vi "MoD Main-Optimize - MS PK.vi"() -> ()   [LabVIEW 2015]
uses:
  <vilib>/silver_ctls/ArrayMatrixCluster/Real Matrix NI_Silver.ctl
  <vilib>/ni845x/ni845x.llb/ni845xControl.ctl
  <vilib>/DAQmx/read.llb/DAQmx Read (Analog 1D DBL NChan 1Samp).vi
  <vilib>/MakerHub/LINX/Public/Peripherals/Analog/Analog Read 1 Chan.vi
  <vilib>/MakerHub/LINX/Public/Peripherals/Analog/Analog Read N Chans.vi
  <vilib>/MakerHub/LINX/Private/Local IO/LinxAnalogRead.vi
  <vilib>/MakerHub/LINX/Public/Utilities/Check Channel.vi
  <vilib>/DAQmx/create/channels.llb/DAQmx Create Channel (AI-Voltage-Basic).vi
  <vilib>/addons/control/pid/pid.llb/PID Control Input Filter (DBL).vi
  <vilib>/DAQmx/miscellaneous.llb/DAQmx Fill In Error Info.vi
  <vilib>/MakerHub/LINX/Private/Utilties/Generate Error.vi
  <vilib>/addons/control/pid/autopid.llb/PID Online Autotuning (Relay Feedback).vi
  <vilib>/Analysis/Matrix/Numeric/Conversions/Array To Matrix - RA2.vi
  <vilib>/ni845x/ni845x.llb/NI-845x Close Device Reference.vi
  <vilib>/addons/control/pid/NI_PID_autopid.lvlib
  <vilib>/addons/control/pid/NI_PID_pid.lvlib
  <vilib>/Analysis/Matrix/NI_Matrix.lvlib
  <vilib>/MakerHub/LINX/LMH-LINX.lvlib
  <vilib>/MakerHub/LINX/Public/Peripherals/Digital/Digital Write 1 Chan.vi
  <instrlib>/Harvard Apparatus/Harvard Apparatus PHD 2000/Harvard Apparatus PHD 2000.lvlib
panel:
  out "MS Array":dbl[](array[numeric]) format="%0.2f"
  out "MS task":refnum<k21>
  out "running?":bool=TRUE
  out "new_reactor_volume":bool[](array[boolean])
  out "new_reactor_length":bool[](array[boolean])
  out "Phase_Sensor_voltage":dbl
  out "P_tot":dbl
  out "stop_xl_write":bool=TRUE
  out "Num_exp_till_pause":i32
  out "Syringe_pump?":bool=TRUE
  out "System Error":bool=TRUE
  out "error out":errorcluster
  out "Pump setpoint(ul/min) 6":dbl format="%#_13g"
  out "Pump setpoint(ul/min) 5":dbl format="%#_13g"
  out "Pump setpoint(ul/min) 4":dbl format="%#_13g"
  out "Pump setpoint(ul/min) 3":dbl format="%#_13g"
  out "Pump setpoint(ul/min) 2":dbl format="%#_13g"
  out "Pump setpoint(ul/min) 1":dbl format="%#_13g"
  out "Volume (ul) 5":dbl format="%#_13g"
  out "Volume (ul) 4":dbl format="%#_13g"
  out "Volume (ul) 3":dbl format="%#_13g"
  out "Volume (ul) 2":dbl format="%#_13g"
  out "Volume (ul) 1":dbl format="%#_13g"
  in  "tau 5":dbl format="%#_13g"
  out "tau 4":dbl format="%#_13g"
  out "tau 3":dbl format="%#_13g"
  out "tau 2":dbl format="%#_13g"
  out "tau 1":dbl format="%#_13g"
  out "Reactor Length":dbl format="%#_13g"
  out "Flowrate Sensor 2":dbl format="%#_13g"
  out "Flowrate Sensor 1":dbl format="%#_13g"
  out "Pressure 2":dbl format="%#_13g"
  out "Pressure 1":dbl format="%#_13g"
  out "Temperature Control 5":bool=TRUE
  out "Temperature Control 4":bool=TRUE
  out "Temperature Control 3":bool=TRUE
  out "Temperature Control 2":bool=TRUE
  out "Temperature Control 1":bool=TRUE
  out "Temperature SP 5":dbl format="%#_g'C"
  out "Temperature SP 4":dbl format="%#_g'C"
  out "Temperature SP 3":dbl format="%#_g'C"
  out "Temperature SP 2":dbl format="%#_g'C"
  out "Temperature SP 1":dbl format="%#_g'C"
  in  "Bay Temperature 5":dbl
  in  "SSR Duration 5":dbl
  in  "SSR Duration 4":dbl
  in  "SSR Duration 3":dbl
  in  "SSR Duration 2":dbl
  in  "SSR Duration 1":dbl
  in  "Total Product Amount":dbl=1.0 format="%#_gml"
  out "Setup Error":bool=TRUE
  out "Error Message":string
  out "ID CTR":i32
  in  "Tab Control":T1(tab)
  out "Reagent pic 5":picture
  in  "reagent name 5":string
  out "Reagent Pic 4":picture
  in  "reagent name 4":string
  out "Reagent Pic 3":picture
  in  "reagent  name 3":string
  in  "Product name":string
  in  "reagent name 1":string="2,5 hexanedione"
  out "Reagent Pic 1":picture
  in  "Vr5":dbl=45.6036 format="%#_guL"
  in  "Vr4":dbl format="%#_guL"
  in  "Vr3":dbl=45.6036 format="%#_guL"
  in  "Vr2":dbl format="%#_guL"
  in  "Vr1":dbl format="%#_guL"
  in  "System decide help Button":bool
  in  "Reaction Scheme Confirm":bool
  in  "Synthesis Route Array":string[][](array[string])=[["2,5 hexanedione", "1", "PhB(OH)2", "", "", ""], ["ethanolamine", "1", "-", "-", "-", "-"], ["", "", "-", "-", "-", "-"], ["", "", "-", "-", "-", "-"], ["", "", "-", "-", "-", "-"], ["", "", "-", "-", "-", "-"]]
  in  "System decide help Button 2":bool
  out "Setup Confirm":bool=TRUE
  in  "BAY 1":u16(ring)=1 items=["               Bypass", "         Heated Reactor", "    Small Heated Reator", "         Cooled Reactor", "      Packed Bed Reactor", "          Photo Reactor", "             Separator"]
  in  "BAY 5":u16(ring) items=["               Bypass", "         Heated Reactor", "    Small Heated Reactor", "         Cooled Reactor", "     Packed Bed Reactor", "         Photo Reactor", "             Separator"]
  in  "BAY 4":u16(ring) items=["                Bypass", "         Heated Reactor", "    Small Heated Reactor", "         Cooled Reactor", "     Packed Bed Reactor", "         Photo Reactor", "             Separator"]
  in  "BAY 3":u16(ring) items=["               Bypass", "         Heated Reactor", "    Small Heated Reactor", "         Cooled Reactor", "     Packed Bed Reactor", "          Photo Reactor", "             Separator"]
  in  "BAY 2":u16(ring) items=["               Bypass", "         Heated Reactor", "    Small Heated Reactor", "         Cooled Reactor", "      Packed Bed Reactor", "          Photo Reactor", "             Separator"]
  out "Reagent Pic 2":picture
  out "Product Pic":picture
  in  "reagent name 2":string="ethanolamine"
  in  "reagent name 6":string
  out "Reagent Pic 6":picture
  in  "System Parameters Help Button":bool
  out "Setup Confirm 2":bool
  in  "System Parameters Confirm Button":bool
  in  "Bay Parameters":T2={"Bay 1 "={"Pump 1 Flowrate"=0.0, "optimize_temp"=TRUE, "optimize_tau"=TRUE, "Run at set flowrate"=FALSE, "Pump 2 Flowrate"=0.0, "Temperature Params"=[40.0, 80.0, 100.0], "pump params 1"=[20.0, 190.0, 325.0], "pump params 2"=[20.0, 190.0, 325.0], "Temperature"=0.0, "Run at set temperature"=FALSE}, "Bay 2 "={"Pump 3 Flowrate"=0.0, "optimize_temp"=FALSE, "optimize_tau"=FALSE, "Run at set flowrate"=FALSE, "Temperature Params"=[40.0, 100.0, 100.0], "Resisdence time params"=[38.03, 347.0, 650.0], "pump_at_ratio"=FALSE, "pump_num_ratio"=0.0, "Temperature"=0.0, "Run at set temperature"=FALSE}, "Bay 3 "={"Pump 4 Flowrate"=100.0, "optimize_temp"=FALSE, "optimize_tau"=FALSE, "Run at set flowrate"=FALSE, "Temperature Params"=[40.0, 100.0, 100.0], "Resisdence time params"=[3.8, 34.7, 0.0], "pump_at_ratio"=FALSE, "pump_num_ratio"=0.2, "Temperature "=100.0, "Run at set temperature"=FALSE}, "Bay 4 "={"Pump 5 Flowrate"=40.0, "Run at set flowrate"=FALSE, "optimize_temp"=FALSE, "optimize_tau"=FALSE, "Resisdence time params"=[10.0, 50.0, 225.0], "Temperature Params"=[40.0, 100.0, 80.0], "pump_at_ratio"=FALSE, "pump_num_ratio"=1.0, "Temperature"=0.0, "Run at set temperature"=FALSE}, "Bay 5 "={"Pump 6 Flowrate"=0.0, "Run at set flowrate"=FALSE, "optimize_temp"=FALSE, "optimize_tau"=FALSE, "Resisdence time params"=[1.0, 5.0, 0.0], "Temperature Params"=[0.0, 0.0, 0.0], "pump_at_ratio"=FALSE, "pump_num_ratio"=0.5, "Temperature"=0.0, "Run at set temperature"=FALSE}, "Excel File Name"="C:\\Users\\Admin\\Dropbox (MIT)\\MoD Files\\Data\\PK_MS080917", "hplc File Name"="C:\\Chem32\\1\\Data\\MOD", "Matlab File"="C:\\Users\\Admin\\Dropbox (MIT)\\MoD Files\\Data\\PK_MS081017", "Syringe for Pump 2?"=TRUE, "Num_conditons_per_wait"=2.0, "Continue from previous optimization?"=FALSE, "Total Number of Experiments 2"=15.0, "Hplc Wait time(min)"=1.0, "increas_decrease_hplc_peak"=TRUE, "Internal Standard?"=TRUE, "ISTD start"=8.0, "ISTD end"=10.0, "hplc_start"=1.75, "hplc_end"=3.0, "throughput_yield"=FALSE} {"Hplc Wait time(min)" format="%#_13g"; "Bay 5"."Temperature Params" format="%#_g'C"; "Bay 4"."Temperature Params" format="%#_g'C"; "Bay 3"."Temperature Params" format="%#_g'C"; "Bay 2"."Temperature Params" format="%#_g'C"; "Bay 1"."Temperature Params" format="%#_g'C"}
  out "System Confirm Not Clicked":string
  out "pause for ms":bool=TRUE
  out "best_exp_num":dbl=1.0
  out "temperature_best":dbl[](array[numeric])
  out "Flowrates(ul/min)_best":dbl[](array[numeric])
  out "System Status":u16(ring)=2 caption="Sy" items=["System  Error", "System Running", "System Standby"]
  out "Current Experiment":dbl=1.0
  out "Total Number of Experiments":dbl=33.0
  out "Phase Sensor Chart":T3(graph)
  out "HPLC Analysis":bool
  out "Equlibrating Temperature":bool
  out "Flushing System":bool
  out "Calculate condition":bool
  out "Temperature 5":dbl format="%#_g'C"
  out "Temperature 4":dbl format="%#_g'C"
  out "Temperature 3":dbl format="%#_g'C"
  out "Temperature 2":dbl format="%#_g'C"
  out "Temperature 1":dbl format="%#_g'C"
  out "Flowrate Chart":T4(graph)
  out "Teperature Chart":T3(graph)
  out "Pump Setpoints Chart":T3(graph)
  out "Pressure Chart":T3(graph)
  out "Optimization_loop_index":i32
  out "curr_wait_time":dbl
  out "total_flush_time":dbl
  out "Temp SS? 5":bool=TRUE
  out "Temp SS? 4":bool=TRUE
  out "Temp SS? 3":bool=TRUE
  out "Temp SS? 2":bool=TRUE
  out "Temp SS? 1":bool=TRUE
  out "System Flushed?":bool
  out "stop_button clicked":bool
  out "MS Signals Chart":dbl[][](graph)
  in  "MS Analog Channel":tag="cDAQ1Mod1/ai0"
  out "experiment history":T5
  in  "Number of System Flushes per condtion":dbl=2.5
  in  "calculate volume 3":bool
  in  "calculate volume 2":bool=TRUE
  in  "calculate volume 1":bool=TRUE
  in  "calculate volume 4":bool
  in  "calculate volume 5":bool
  in  "Extra system dead volume":dbl format="%#_gul"
  in  "new reactor length? 1":bool
  in  "tube_length(in)":dbl[](array[numeric])=[188.0, 188.0, 10.0, 10.0, 10.0]
  out "Pause Before Analysis":bool
  out "Chiller COMM Port":bool
  out "Arduino COMM Port 2":bool
  out "Temperature Sensor COMM Port":bool
  out "Flow Rate":bool
  out "Pressure":bool
  out "Pump COMM Port":bool
  in  "COMM Port :: Milligat Pumps":refnum<visa-resource-name>="COM8"
  in  "Arduino COMM Port":refnum<visa-resource-name>="COM7"
  in  "Sample Valve COMM::Port":refnum<visa-resource-name>="COM10"
  in  "COMM Port:: Harvard Syringe Pump":refnum<visa-resource-name>="COM13"
  in  "tube_id(in)":enum16{".01", ".02", ".03", ".04"}[](array[ring])=[enum.".03", enum.".03", enum.".03", enum.".03", enum.".03"]
  out "Total System Resisdence Time(min)":dbl
  in  "Debug_run_button":bool
  in  "new reactor length? 2":bool
  in  "new reactor length? 3":bool
  in  "new reactor length? 4":bool
  in  "new reactor length? 5":bool
  in  "IR Sensor Device":T6="USB0::0x3923::0x7514::01B3FF21::RAW"
  out "Stop":bool=TRUE
  in  "Run_Stop_cluster":T7
  # "Molecules on Demand"
  # "Synthetic Route"
  # "5"
  # "6"
  # "4"
  # "Product"
  # "1"
  # "2"
  # "3"
  # "Reagent List"
  # "Concentration(M)"
  # "Molecule"
  # "1"
  # "1"
  # "2"
  # "2"
  # "3"
  # "3"
  # "4"
  # "4"
  # "5"
  # "6"
  # "5"
  # "6"
  # "Product"
  # "Reactor Volume:"
  # "Optimization Parameters"
  # "Pause after"
  # "Experiments"
  # "Optimize for"
  # "to"
  # "of HPLC Peak from"
  # "from"
  # "to"
  # "min"
  # "min"
  # "HPLC runtime"
  # "# Iterations"
  # "Reporting"
  # "Excel Output File Name"
  # "HPLC File Path"
  # "MATLAB File Path"
  # "Temperature"
  # "Flowrate(ul/min)"
  # "Lower Bound"
  # "Upper Bound"
  # "Optimize?"
  # "-or-"
  # "Run at"
  # "times incoming flow"
  # "Setpoint"
  # "Temperature"
  # "Flowrate(ul/min)"
  # "Lower Bound"
  # "Upper Bound"
  # "Optimize?"
  # "-or-"
  # "Run at"
  # "times incoming flow"
  # "Setpoint"
  # "Temperature"
  # "Flowrate(ul/min)"
  # "Lower Bound"
  # "Upper Bound"
  # "Optimize?"
  # "-or-"
  # "Run at"
  # "times incoming flow"
  # "Setpoint"
  # "Temperature"
  # "Flowrate 3 (ul/min)"
  # "Lower Bound"
  # "Upper Bound"
  # "Optimize?"
  # "-or-"
  # "Run at"
  # "times incoming flow"
  # "Setpoint"
  # "Temperature"
  # "Flowrate 1(ul/min)"
  # "Flowrate 2(ul/min)"
  # "Lower Bound"
  # "Upper Bound"
  # "Optimize?"
  # "Setpoint"
  # "Pressure (psi)"
  # "System Status"
  # "Temperature('C)"
  # "BAY"
  # "1"
  # "2"
  # "3"
  # "4"
  # "5"
  # "Pump Flowrate Setpoint(ul/min)"
  # "Flowrate (ul/min)"
  # "Phase Sensor"
  # "Current Experiment"
  # "MS Chart"
  # "Temperature('C)"
  # "Flowrate(ul/min)"
  # "Exp"
  # "Current Best Condition"
  # "Time to reach steady state:"
  # "Current Wait Time:"
  # "Experimental Steps"
  # "Calculated New Conditions"
  # "Steady State"
  # "Analyzed HPLC"
  # "Equilibrated Temperature"
  # "Tube Length (cm)"
  # "Bay"
  # "Tube ID (in)"
  # "Calculate Volume"
  # "Use new tube length"
  # "1."
  # "2."
  # "3."
  # "4."
  # "5."
  # "Reactor Lengths\n*Heated Reactor - 188cm * Small Reactor - 99cm * Bypass - 10cm * Separator - *"
  # "All Experimental Data"
  # "P1"
  # "P2"
  # "P3"
  # "P4"
  # "P5"
  # "P6"
  # "T1"
  # "T2"
  # "T3"
  # "T4"
  # "T5"
  # "Obj_fun"
  # "HPLC_Data"
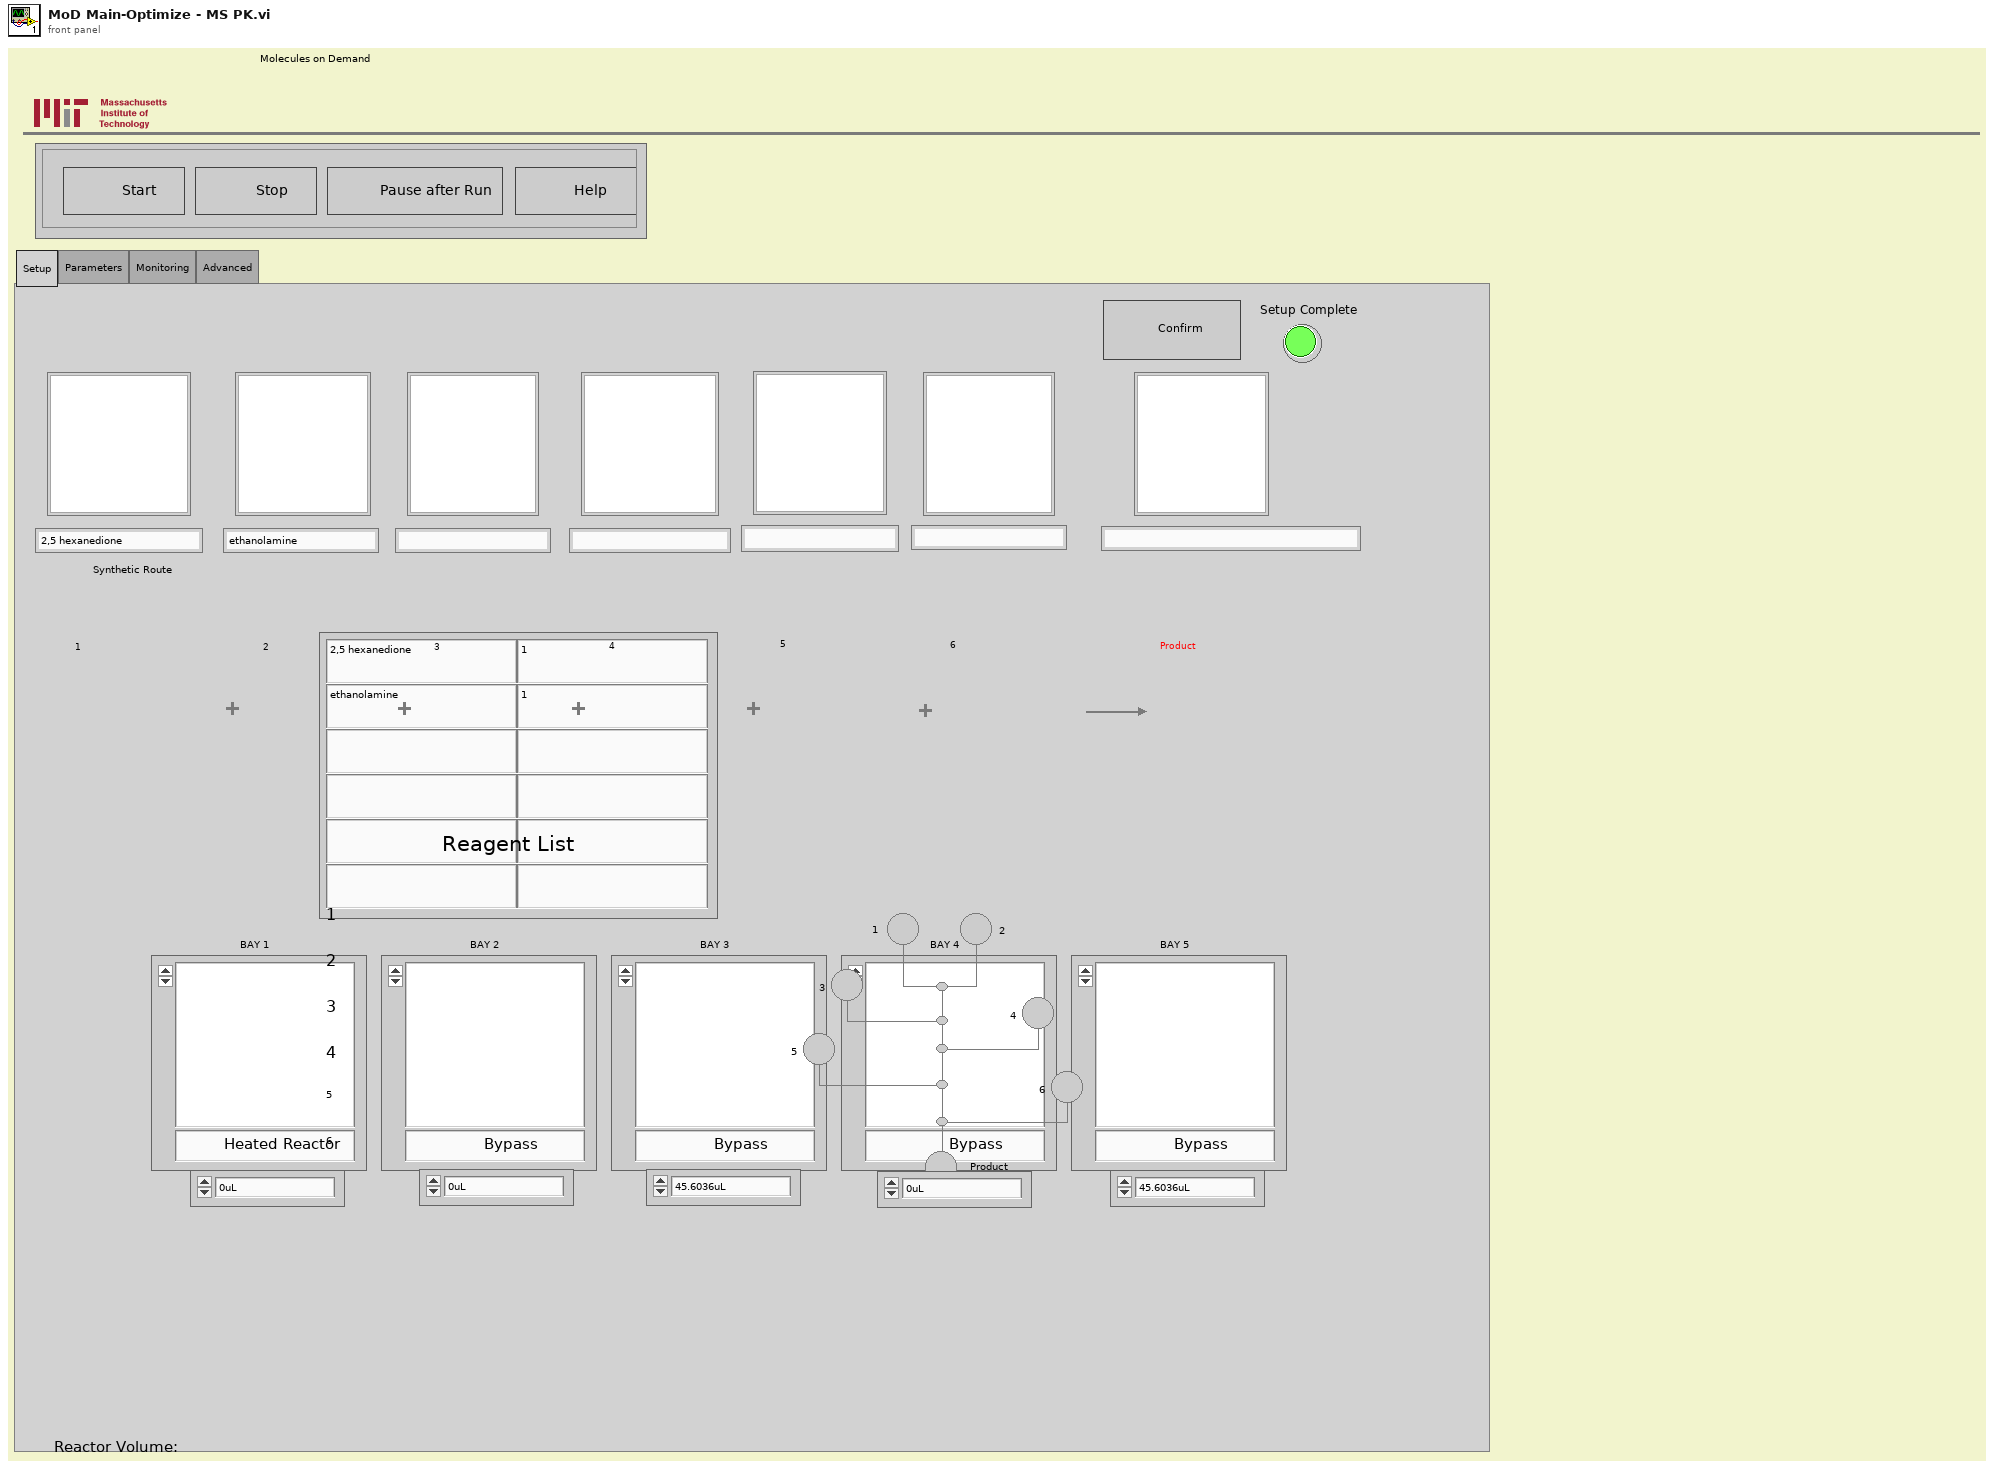
[diagram p1: front panel]
types:
  T1 = enum32{"Setup", "Parameters", "Monitoring", "Advanced"}
  T2 = cluster{"Bay 1 ":cluster{"Pump 1 Flowrate":dbl, "optimize_temp":bool, "optimize_tau":bool, "Run at set flowrate":bool, "Pump 2 Flowrate":dbl, "Temperature Params":dbl[], "pump params 1":dbl[], "pump params 2":dbl[], "Temperature":dbl, "Run at set temperature":bool}, "Bay 2 ":cluster{"Pump 3 Flowrate":dbl, "optimize_temp":bool, "optimize_tau":bool, "Run at set flowrate":bool, "Temperature Params":dbl[], "Resisdence time params":dbl[], "pump_at_ratio":bool, "pump_num_ratio":dbl, "Temperature":dbl, "Run at set temperature":bool}, "Bay 3 ":cluster{"Pump 4 Flowrate":dbl, "optimize_temp":bool, "optimize_tau":bool, "Run at set flowrate":bool, "Temperature Params":dbl[], "Resisdence time params":dbl[], "pump_at_ratio":bool, "pump_num_ratio":dbl, "Temperature ":dbl, "Run at set temperature":bool}, "Bay 4 ":cluster{"Pump 5 Flowrate":dbl, "Run at set flowrate":bool, "optimize_temp":bool, "optimize_tau":bool, "Resisdence time params":dbl[], "Temperature Params":dbl[], "pump_at_ratio":bool, "pump_num_ratio":dbl, "Temperature":dbl, "Run at set temperature":bool}, "Bay 5 ":cluster{"Pump 6 Flowrate":dbl, "Run at set flowrate":bool, "optimize_temp":bool, "optimize_tau":bool, "Resisdence time params":dbl[], "Temperature Params":dbl[], "pump_at_ratio":bool, "pump_num_ratio":dbl, "Temperature":dbl, "Run at set temperature":bool}, "Excel File Name":string, "hplc File Name":string, "Matlab File":string, "Syringe for Pump 2?":bool, "Num_conditons_per_wait":dbl, "Continue from previous optimization?":bool, "Total Number of Experiments 2":dbl, "Hplc Wait time(min)":dbl, "increas_decrease_hplc_peak":bool, "Internal Standard?":bool, "ISTD start":dbl, "ISTD end":dbl, "hplc_start":dbl, "hplc_end":dbl, "throughput_yield":bool}
  T3 = cluster{"[0]":dbl, "[1]":dbl, "[2]":dbl, "[3]":dbl, "[4]":dbl, "[5]":dbl, "[6]":dbl, "[7]":dbl, "[8]":dbl}
  T4 = cluster{"[0]":i32, "[1]":i32, "[2]":i32, "[3]":i32, "[4]":i32, "[5]":i32, "[6]":i32, "[7]":i32, "[8]":i32}
  T5 = typedef "Real Matrix NI_Silver.ctl" = dbl[][]
  T6 = typedef "ni845xControl.ctl" = refnum<k21>
  T7 = cluster{"Stop":bool, "Run":bool, "Stop Run Button":bool, "Help Button":bool}
  T8 = cluster{"Proportional gain Kc":dbl, "Integral time Ti (sec)":dbl, "Derivative time Ti (sec)":dbl}
  T9 = cluster{"type of controller":enum16{"P", "PI", "PID"}, "relay cycles":i32, "relay amplitude":dbl, "control specifications":enum16{"Fast", "Normal", "Slow"}, "PV noise level":dbl}
  T10 = typedef "LMH-LINX.lvlib/LINX Ref.ctl" = cluster{"IO":T11, "Interface":T12, "LINX Device Config":T13}
  T11 = typedef "LMH-LINX.lvlib/Platform.ctl" = enum16{"Remote", "Local"}
  T12 = typedef "LMH-LINX.lvlib/Interface.ctl" = enum16{"Serial", "TCP"}
  T13 = typedef "LMH-LINX.lvlib/Device.lvlib/LINX Device Config.ctl" = cluster{"Interface":T12, "COM Port":refnum<visa-resource-name>, "TCP Configuration":T14, "Device Family":u8, "Device ID":u8, "Device Name":string, "TCP Ref":refnum<k5>, "Channels":T15}
  T14 = typedef "LMH-LINX.lvlib/Device.lvlib/TCP Config.ctl" = cluster{"IP Address":string, "Port":u16}
  T15 = typedef "LMH-LINX.lvlib/Channels.ctl" = cluster{"DI":u8[], "DO":u8[], "AI":u8[], "AO":u8[], "PWM":u8[], "QE":u8[], "UART":u8[], "I2C 2":u8[], "SPI":u8[], "CAN":u8[], "Servo":u8[], "AI Ref (V)":dbl, "AI Resolution (Bits)":u8, "AO Ref (V)":dbl, "AO Resolution (Bits)":u8}
  T16 = typedef "imagedata.ctl" = cluster{"image type":i32, "image depth":i32, "image":u8[], "mask":u8[], "colors":u32[], "Rectangle":cluster{"left":i16, "top":i16, "right":i16, "bottom":i16}}
  T17 = cluster{"proportional gain (Kc)":dbl, "integral time (Ti, min)":dbl, "derivative time (Td, min)":dbl}
  T18 = typedef "NI_Matrix.lvlib/RealMatrix.ctl" = dbl[][]
  T19 = enum16{"Left Button", "Center Button", "Right Button", "Window Close"}
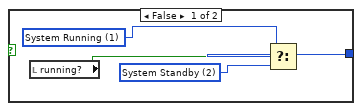
[diagram p3: hidden frame]
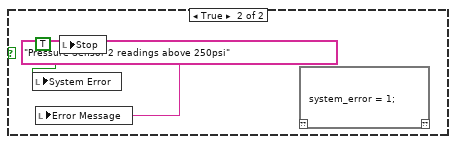
[diagram p4: hidden frame]
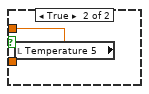
[diagram p6: hidden frame]
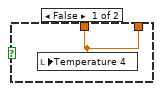
[diagram p7: hidden frame]
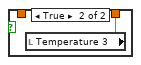
[diagram p8: hidden frame]
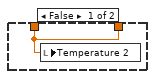
[diagram p9: hidden frame]
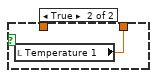
[diagram p10: hidden frame]
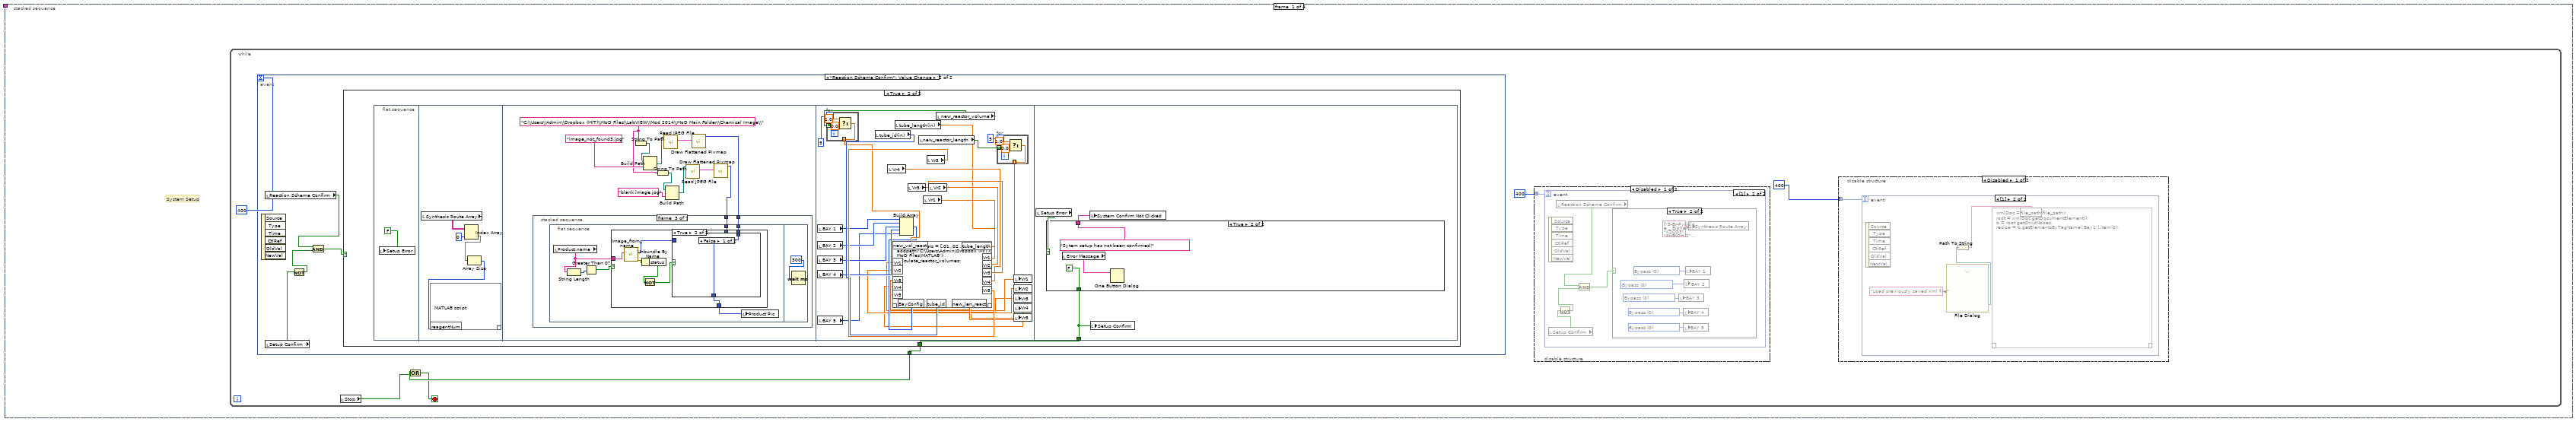
[diagram p11: hidden frame]
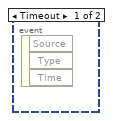
[diagram p12: hidden frame]
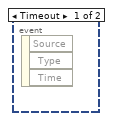
[diagram p14: hidden frame]
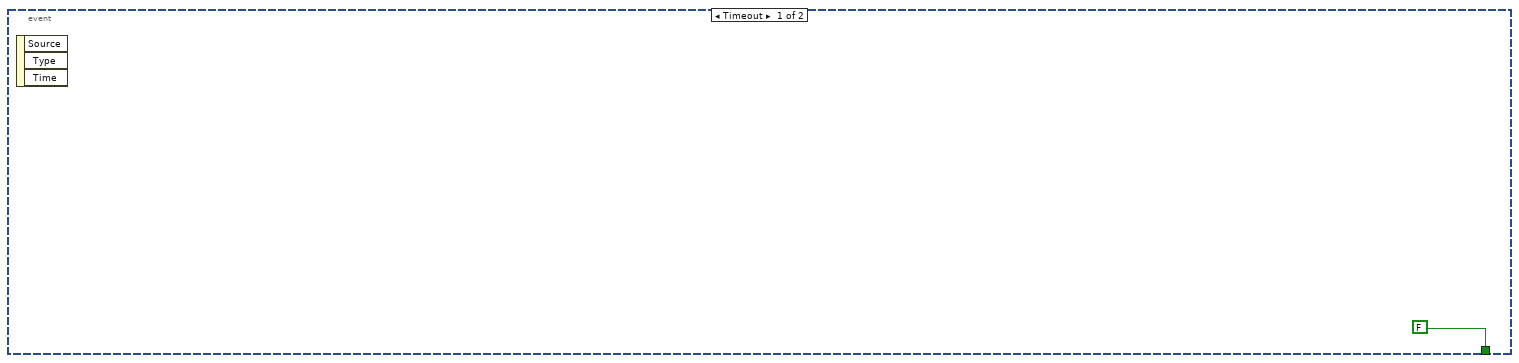
[diagram p17: hidden frame]
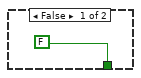
[diagram p18: hidden frame]
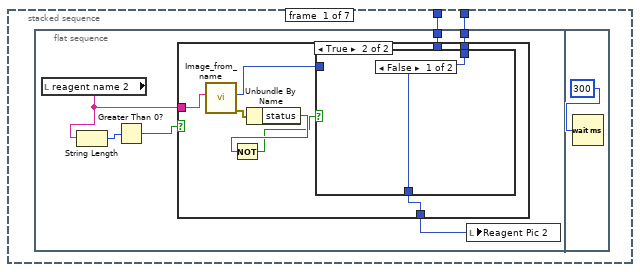
[diagram p19: hidden frame]
diagram:
  # "Assume User always uses the first bay first"
  n1 = flat-sequence {
    tunnel: ["COMM Port :: Milligat Pumps"] -> w9
    tunnel: ["Arduino COMM Port"] -> w8
    tunnel: [w13] -> w5
    tunnel: ["Bay Parameters"] -> w4
    tunnel: [w61] -> w10
    tunnel: w9 -> [w61]
    tunnel: w8 -> [w49]
    tunnel: [w55] -> w7
    tunnel: [w53] -> w6
    tunnel: w5 -> [w53]
    tunnel: w4 -> [w51]
    tunnel: [w48] -> w3
    tunnel: w10 -> [w67]
    tunnel: w7 -> [w66]
    tunnel: w6 -> [w64]
    tunnel: w3 -> [w62]
    tunnel: [w62] -> w1
    tunnel: [w1358] -> w2
    tunnel: w1 -> [w1358]
    tunnel: w2 -> [w1359]
    frame #0 {
      w37 = FALSE ("Equlibrating Temperature")
      n2 = call-poly <vilib>:"DAQmx Create Virtual Channel.vi"("physical channels"="MS Analog Channel") -> ("task out"=→"MS task":refnum<k21>)  [unwired: 13 in, 1 out]
      n3 = script code="TempArr1=[23 23 23 23 23 23 23 23 23 23]';\nTempArr2=[23 23 23 23 23 23 23 23 23 23]';\nTempArr3=[23 23 23 23 23 23 23 23 23 23]';\nTempArr4=[23 23 23 23 23 23 23 23 23 23]';\nTempArr5=[23 23 23 23 23 23 23 23 23 23]';\ntemp_error1 =0;\ntemp_error2 =0;\ntemp_error3 =0;\ntemp_error4 =0;\ntemp_error5 =0;\ntemp_check1 = 0;\ntemp_check2 = 0;\ntemp_check3 = 0;\ntemp_check4 = 0;\ntemp_check5 = 0;\nT1=23;\nT2=23;\nT3=23;\nT4=23;\nT5=23;"() -> ()  [unwired: 1 in, 1 out]
      n4 = Build Array("calculate volume 1", "calculate volume 2", "calculate volume 3", "calculate volume 4", "calculate volume 5") -> (→"new_reactor_volume":bool[])
      n5 = Build Array("new reactor length? 1", "new reactor length? 2", "new reactor length? 3", "new reactor length? 4", "new reactor length? 5") -> (→"new_reactor_length":bool[])
      n6 = call <vilib>:"Initialize.vi"("VISA IN"="COMM Port:: Harvard Syringe Pump") -> ("VISA OUT"=w13:refnum<visa-resource-name>)  [unwired: 13 in, 1 out]
      "Stop" <- FALSE ("Stop")
      "ID CTR" <- 0
      "Setup Confirm" <- FALSE ("Setup Confirm")
      "Error Message" <- "System shutdown sucessfully. No errors to report." ("Error Message")
      "Setup Error" <- FALSE ("Setup Error")
      "Reactor Length" <- 10.5
      "System Error" <- FALSE ("System Error")
      "Num_exp_till_pause" <- 0 ("Num_exp_till_pause")
      "Equlibrating Temperature" <- w37
      "Calculate condition" <- w37
      "Flushing System" <- w37
      "HPLC Analysis" <- w37
      "stop_xl_write" <- FALSE ("stop_xl_write")
      "Pump setpoint(ul/min) 1" <- 0.0 ("Pump setpoint(ul/min) 1")
      "Pump setpoint(ul/min) 2" <- 0.0 ("Pump setpoint(ul/min) 2")
      "Pump setpoint(ul/min) 4" <- 0.0 ("Pump setpoint(ul/min) 4")
      "Pump setpoint(ul/min) 6" <- 0.0 ("Pump setpoint(ul/min) 6")
      "Pump setpoint(ul/min) 3" <- 0.0 ("Pump setpoint(ul/min) 3")
      "Pump setpoint(ul/min) 5" <- 0.0 ("Pump setpoint(ul/min) 5")
      "Setup Confirm 2" <- FALSE ("Setup Confirm 2")
      "running?" <- FALSE ("running?")
    }
    frame #1 {
      w50 = FALSE
      w60 = 23
      (unwired) path "C:/Users/User1/Documents/Lab/MoD/Images"
      n7 = disable-structure shown="Disabled" {
        frame Disabled {
          n8 = local read "BAY 2"() -> ()  [unwired: 1 out]
          n9 = local read "BAY 3"() -> ()  [unwired: 1 out]
          n10 = local read "BAY 4"() -> ()  [unwired: 1 out]
          n11 = local read "BAY 5"() -> ()  [unwired: 1 out]
          n12 = local read "BAY 1"() -> ()  [unwired: 1 out]
        }
        frame Enabled {
        }
      }
      n13 = local write "Debug_run_button"(TRUE) -> ()
      n14 = call <vilib>:"Initialize.vi"("Serial Port"=w49) -> ("LINX Resource"=w48:T10)  [unwired: 8 in, 2 out]
      n15 = local write "System Parameters Confirm Button"(w50) -> ()
      n16 = local write "Setup Confirm 2"(w50) -> ()
      n17 = Unbundle By Name(w51) -> ("Syringe for Pump 2?"=→"Syringe_pump?":bool)
      n18 = local write "Temperature 1"(w60) -> ()
      n19 = local write "Temperature 2"(w60) -> ()
      n20 = local write "Temperature 3"(w60) -> ()
      n21 = local write "Temperature 4"(w60) -> ()
      n22 = local write "Temperature 5"(w60) -> ()
      n23 = local write "Temperature SP 1"(w60) -> ()
      n24 = local write "Temperature SP 2"(w60) -> ()
      n25 = local write "Temperature SP 3"(w60) -> ()
      n26 = local write "Temperature SP 4"(w60) -> ()
      n27 = local write "Temperature SP 5"(w60) -> ()
      n28 = Current VI's Path() -> (path=w59:path)
      n29 = Strip Path(path=w59) -> (stripped path=w57:path)  [unwired: 1 out]
      n30 = Strip Path(path=w57) -> (stripped path=w56:path)  [unwired: 1 out]
      n31 = Build Path(base path=w56, name or relative path="MATLAB") -> (appended path=w55:path)
    }
    frame #2 {
      # "Main Help Dialog Popup"
      n32 = while {
        stop <- w1352 stop-if-true
        n33 = event shown="[6] \"Run_Stop_cluster.Run\": Value Change" {
          selector: _ -> [_ _ _ _ _ _ _]
          dyn-events: _ -> [_ _ _ _ _ _ _]
          timeout: 100 -> [_ _ _ _ _ _ _]
          event Timeout {
            n34 = event-data() -> ()  [unwired: 1 in, 3 out]
          }
          event "Run_Stop_cluster.Help Button": Value Change {
            n35 = local read "Run_Stop_cluster"() -> (w1355:T7)
            n36 = event-data() -> ()  [unwired: 1 in, 4 out]
            n37 = Unbundle By Name(w1355) -> ("Help Button"=w1354:bool)
            n38 = case shown="True" w1354 {
              frame False {
              }
              frame True {
                n39 = call "help.vi"() -> ()  [unwired: 11 in]
              }
            }
          }
          event "System decide help Button": Value Change {
            n40 = event-data() -> ()  [unwired: 1 in, 5 out]
            n41 = call "help_synthesis_man-auto_instructions.vi"() -> ()  [unwired: 12 in]
          }
          event "System Parameters Help Button": Value Change {
            n42 = event-data() -> ()  [unwired: 1 in, 5 out]
            n43 = call "help_parameters_setup.vi"() -> ()  [unwired: 12 in]
          }
          event "System decide help Button 2": Value Change {
            n44 = event-data() -> ()  [unwired: 1 in, 5 out]
            n45 = call "help_synthesis_route_instructions.vi"() -> ()  [unwired: 12 in]
          }
          event "Run_Stop_cluster.Stop": Value Change {
            n46 = event-data() -> ()  [unwired: 1 in, 5 out]
            n47 = local write "Stop"(TRUE) -> ()
          }
          event "Run_Stop_cluster.Run": Value Change {
            n48 = event-data() -> ()  [unwired: 1 in, 5 out]
            n49 = local write "running?"(TRUE) -> ()
          }
        }
        n50 = local read "Stop"() -> (w1352:bool)
      }
      n51 = stacked-sequence {
        tunnel: w67 -> [_ _ _ _]
        tunnel: w66 -> [_ w431 _ _]
        tunnel: w64 -> [_ _ _ w598]
        tunnel: w62 -> [_ _ _ w596]
        frame #0 {
          # "System Setup"
          n52 = while {
            stop <- w206 stop-if-true
            n53 = event shown="[1] \"Reaction Scheme Confirm\": Value Change" {
              selector: _ -> [_ _]
              dyn-events: _ -> [_ _]
              timeout: 400 -> [_ _]
              tunnel: [FALSE w226] -> w208
              event Timeout {
                n54 = event-data() -> ()  [unwired: 1 in, 3 out]
              }
              event "Reaction Scheme Confirm": Value Change {
                n55 = event-data() -> ()  [unwired: 1 in, 6 out]
                n56 = local read "Reaction Scheme Confirm"() -> (w230:bool)
                n57 = local read "Setup Confirm"() -> (w228:bool)
                n58 = Not(x=w228) -> (.not. x?=w227:bool)
                n59 = And(x=w230, y=w227) -> (x .and. y?=w229:bool)
                n60 = case shown="True" w229 {
                  tunnel: [FALSE w232] -> w226
                  frame False {
                  }
                  frame True {
                    n61 = flat-sequence {
                      tunnel: [w421] -> w232
                      frame #0 {
                        n62 = local write "Setup Error"(FALSE) -> ()
                      }
                      frame #1 {
                        n63 = local read "Synthesis Route Array"() -> (w236:string[][])
                        n64 = Index Array(array=w236, index (col)=0 ("disabled index (col)")) -> (element=w234:string[])  [unwired: 1 in]
                        n65 = Array Size(array=w234) -> (size(s)=w237:i32)
                        n66 = script code="MATLAB script"("reagentNum"=w237) -> ()  [unwired: 1 in, 1 out]
                      }
                      frame #2 {
                        w240 = "C:\\Users\\Admin\\Dropbox (MIT)\\MoD Files\\LabVIEW\\Mod 2014\\MoD Main Folder\\Chemical Image\\" ("string")
                        n67 = String To Path(string=w240) -> (path=w246:path)
                        n68 = Build Path(base path=w246, name or relative path="image_not_found3.jpg") -> (appended path=w245:path)
                        n69 = String To Path(string=w240) -> (path=w243:path)
                        n70 = call <vilib>:"Read JPEG File.vi"("path to JPEG file"=w245) -> ("image data"=w248:T16)  [unwired: 1 in, 9 out]
                        n71 = Build Path(base path=w243, name or relative path="blank image.jpg") -> (appended path=w241:path)
                        n72 = call <vilib>:"Read JPEG File.vi"("path to JPEG file"=w241) -> ("image data"=w244:T16)  [unwired: 1 in, 9 out]
                        n73 = call <vilib>:"Draw Flattened Pixmap.vi"("image data"=w248) -> ("new picture"=w239:picture)  [unwired: 3 in, 5 out]
                        n74 = call <vilib>:"Draw Flattened Pixmap.vi"("image data"=w244) -> ("new picture"=w238:picture)  [unwired: 3 in, 5 out]
                        n75 = stacked-sequence {
                          tunnel: w239 -> [w250 w270 w290 w310 w330 w349 w369]
                          tunnel: w238 -> [w249 w269 w289 w309 w329 w350 w370]
                          frame #0 {
                            n76 = flat-sequence {
                              tunnel: w250 -> [w256]
                              tunnel: w249 -> [w254]
                              frame #0 {
                                n77 = local read "reagent name 2"() -> (w252:string)
                                n78 = String Length(string=w252) -> (length=w255:i32)
                                n79 = Greater Than 0?(x=w255) -> (x > 0?=w253:bool)
                                n80 = case shown="True" w253 {
                                tunnel: w256 -> [_ w262]
                                tunnel: w254 -> [w257 _]
                                tunnel: [w257 w261] -> w251
                                tunnel: w252 -> [_ w260]
                                frame False {
                                }
                                frame True {
                                n81 = call "Image_from_name.vi"("Chemical Name"=w260) -> ("error out"=w263:errorcluster, "Downloaded Picture"=w264:picture)  [unwired: 8 in, 1 out]
                                n82 = Unbundle By Name(w263) -> ("status"=w259:bool)
                                n83 = Not(x=w259) -> (.not. x?=w258:bool)
                                n84 = case shown="False" w258 {
                                tunnel: w264 -> [_ w267]
                                tunnel: [w265 w266] -> w261
                                tunnel: w262 -> [w265 _]
                                frame False {
                                }
                                frame True {
                                n85 = call <vilib>:"Draw Flattened Pixmap.vi"("picture"=w267) -> ("new picture"=w266:picture)  [unwired: 8 in]
                                }
                                }
                                }
                                }
                                n86 = local write "Reagent Pic 2"(w251) -> ()
                              }
                              frame #1 {
                                n87 = Wait (ms)(milliseconds to wait=300) -> ()  [unwired: 1 out]
                              }
                            }
                          }
                          frame #1 {
                            n88 = flat-sequence {
                              tunnel: w270 -> [w276]
                              tunnel: w269 -> [w274]
                              frame #0 {
                                n89 = local read "reagent name 1"() -> (w271:string)
                                n90 = String Length(string=w271) -> (length=w275:i32)
                                n91 = Greater Than 0?(x=w275) -> (x > 0?=w273:bool)
                                n92 = case shown="True" w273 {
                                tunnel: w276 -> [_ w282]
                                tunnel: w274 -> [w277 _]
                                tunnel: [w277 w281] -> w272
                                tunnel: w271 -> [_ w280]
                                frame False {
                                }
                                frame True {
                                n93 = call "Image_from_name.vi"("Chemical Name"=w280) -> ("error out"=w283:errorcluster, "Downloaded Picture"=w284:picture)  [unwired: 8 in, 1 out]
                                n94 = Unbundle By Name(w283) -> ("status"=w279:bool)
                                n95 = Not(x=w279) -> (.not. x?=w278:bool)
                                n96 = case shown="True" w278 {
                                tunnel: w284 -> [_ w287]
                                tunnel: [w285 w286] -> w281
                                tunnel: w282 -> [w285 _]
                                frame False {
                                }
                                frame True {
                                n97 = call <vilib>:"Draw Flattened Pixmap.vi"("picture"=w287) -> ("new picture"=w286:picture)  [unwired: 8 in]
                                }
                                }
                                }
                                }
                                n98 = local write "Reagent Pic 1"(w272) -> ()
                              }
                              frame #1 {
                                n99 = Wait (ms)(milliseconds to wait=300) -> ()  [unwired: 1 out]
                              }
                            }
                          }
                          frame #2 {
                            n100 = flat-sequence {
                              tunnel: w290 -> [w296]
                              tunnel: w289 -> [w294]
                              frame #0 {
                                n101 = local read "Product name"() -> (w291:string)
                                n102 = String Length(string=w291) -> (length=w295:i32)
                                n103 = Greater Than 0?(x=w295) -> (x > 0?=w293:bool)
                                n104 = case shown="True" w293 {
                                tunnel: w296 -> [_ w302]
                                tunnel: w294 -> [w297 _]
                                tunnel: [w297 w301] -> w292
                                tunnel: w291 -> [_ w300]
                                frame False {
                                }
                                frame True {
                                n105 = call "Image_from_name.vi"("Chemical Name"=w300) -> ("error out"=w303:errorcluster, "Downloaded Picture"=w304:picture)  [unwired: 8 in, 1 out]
                                n106 = Unbundle By Name(w303) -> ("status"=w298:bool)
                                n107 = Not(x=w298) -> (.not. x?=w299:bool)
                                n108 = case shown="False" w299 {
                                tunnel: w304 -> [_ w307]
                                tunnel: [w305 w306] -> w301
                                tunnel: w302 -> [w305 _]
                                frame False {
                                }
                                frame True {
                                n109 = call <vilib>:"Draw Flattened Pixmap.vi"("picture"=w307) -> ("new picture"=w306:picture)  [unwired: 8 in]
                                }
                                }
                                }
                                }
                                n110 = local write "Product Pic"(w292) -> ()
                              }
                              frame #1 {
                                n111 = Wait (ms)(milliseconds to wait=300) -> ()  [unwired: 1 out]
                              }
                            }
                          }
                          frame #3 {
                            n112 = flat-sequence {
                              tunnel: w310 -> [w316]
                              tunnel: w309 -> [w314]
                              frame #0 {
                                n113 = local read "reagent name 6"() -> (w311:string)
                                n114 = String Length(string=w311) -> (length=w315:i32)
                                n115 = Greater Than 0?(x=w315) -> (x > 0?=w313:bool)
                                n116 = case shown="True" w313 {
                                tunnel: w316 -> [_ w322]
                                tunnel: w314 -> [w317 _]
                                tunnel: [w317 w321] -> w312
                                tunnel: w311 -> [_ w320]
                                frame False {
                                }
                                frame True {
                                n117 = call "Image_from_name.vi"("Chemical Name"=w320) -> ("error out"=w323:errorcluster, "Downloaded Picture"=w324:picture)  [unwired: 8 in, 1 out]
                                n118 = Unbundle By Name(w323) -> ("status"=w318:bool)
                                n119 = Not(x=w318) -> (.not. x?=w319:bool)
                                n120 = case shown="False" w319 {
                                tunnel: w324 -> [_ w327]
                                tunnel: [w325 w326] -> w321
                                tunnel: w322 -> [w325 _]
                                frame False {
                                }
                                frame True {
                                n121 = call <vilib>:"Draw Flattened Pixmap.vi"("picture"=w327) -> ("new picture"=w326:picture)  [unwired: 8 in]
                                }
                                }
                                }
                                }
                                n122 = local write "Reagent Pic 6"(w312) -> ()
                              }
                              frame #1 {
                                n123 = Wait (ms)(milliseconds to wait=300) -> ()  [unwired: 1 out]
                              }
                            }
                          }
                          frame #4 {
                            n124 = flat-sequence {
                              tunnel: w330 -> [w336]
                              tunnel: w329 -> [w334]
                              frame #0 {
                                n125 = local read "reagent name 5"() -> (w331:string)
                                n126 = String Length(string=w331) -> (length=w335:i32)
                                n127 = Greater Than 0?(x=w335) -> (x > 0?=w333:bool)
                                n128 = case shown="True" w333 {
                                tunnel: w336 -> [_ w342]
                                tunnel: w334 -> [w337 _]
                                tunnel: [w337 w341] -> w332
                                tunnel: w331 -> [_ w340]
                                frame False {
                                }
                                frame True {
                                n129 = call "Image_from_name.vi"("Chemical Name"=w340) -> ("error out"=w343:errorcluster, "Downloaded Picture"=w344:picture)  [unwired: 8 in, 1 out]
                                n130 = Unbundle By Name(w343) -> ("status"=w338:bool)
                                n131 = Not(x=w338) -> (.not. x?=w339:bool)
                                n132 = case shown="False" w339 {
                                tunnel: w344 -> [_ w347]
                                tunnel: [w345 w346] -> w341
                                tunnel: w342 -> [w345 _]
                                frame False {
                                }
                                frame True {
                                n133 = call <vilib>:"Draw Flattened Pixmap.vi"("picture"=w347) -> ("new picture"=w346:picture)  [unwired: 8 in]
                                }
                                }
                                }
                                }
                                n134 = local write "Reagent pic 5"(w332) -> ()
                              }
                              frame #1 {
                                n135 = Wait (ms)(milliseconds to wait=300) -> ()  [unwired: 1 out]
                              }
                            }
                          }
                          frame #5 {
                            n136 = flat-sequence {
                              tunnel: w350 -> [w354]
                              tunnel: w349 -> [w353]
                              frame #0 {
                                n137 = local read "reagent name 4"() -> (w351:string)
                                n138 = String Length(string=w351) -> (length=w356:i32)
                                n139 = Greater Than 0?(x=w356) -> (x > 0?=w355:bool)
                                n140 = case shown="True" w355 {
                                tunnel: w353 -> [_ w362]
                                tunnel: w354 -> [w357 _]
                                tunnel: [w357 w361] -> w352
                                tunnel: w351 -> [_ w360]
                                frame False {
                                }
                                frame True {
                                n141 = call "Image_from_name.vi"("Chemical Name"=w360) -> ("error out"=w363:errorcluster, "Downloaded Picture"=w364:picture)  [unwired: 8 in, 1 out]
                                n142 = Unbundle By Name(w363) -> ("status"=w358:bool)
                                n143 = Not(x=w358) -> (.not. x?=w359:bool)
                                n144 = case shown="False" w359 {
                                tunnel: w364 -> [_ w367]
                                tunnel: [w365 w366] -> w361
                                tunnel: w362 -> [w365 _]
                                frame False {
                                }
                                frame True {
                                n145 = call <vilib>:"Draw Flattened Pixmap.vi"("picture"=w367) -> ("new picture"=w366:picture)  [unwired: 8 in]
                                }
                                }
                                }
                                }
                                n146 = local write "Reagent Pic 4"(w352) -> ()
                              }
                              frame #1 {
                                n147 = Wait (ms)(milliseconds to wait=300) -> ()  [unwired: 1 out]
                              }
                            }
                          }
                          frame #6 {
                            n148 = flat-sequence {
                              tunnel: w370 -> [w374]
                              tunnel: w369 -> [w373]
                              frame #0 {
                                n149 = local read "reagent  name 3"() -> (w371:string)
                                n150 = String Length(string=w371) -> (length=w376:i32)
                                n151 = Greater Than 0?(x=w376) -> (x > 0?=w375:bool)
                                n152 = case shown="True" w375 {
                                tunnel: w373 -> [_ w382]
                                tunnel: w374 -> [w377 _]
                                tunnel: [w377 w381] -> w372
                                tunnel: w371 -> [_ w380]
                                frame False {
                                }
                                frame True {
                                n153 = call "Image_from_name.vi"("Chemical Name"=w380) -> ("error out"=w383:errorcluster, "Downloaded Picture"=w384:picture)  [unwired: 8 in, 1 out]
                                n154 = Unbundle By Name(w383) -> ("status"=w378:bool)
                                n155 = Not(x=w378) -> (.not. x?=w379:bool)
                                n156 = case shown="False" w379 {
                                tunnel: w384 -> [_ w387]
                                tunnel: [w385 w386] -> w381
                                tunnel: w382 -> [w385 _]
                                frame False {
                                }
                                frame True {
                                n157 = call <vilib>:"Draw Flattened Pixmap.vi"("picture"=w387) -> ("new picture"=w386:picture)  [unwired: 8 in]
                                }
                                }
                                }
                                }
                                n158 = local write "Reagent Pic 3"(w372) -> ()
                              }
                              frame #1 {
                                n159 = Wait (ms)(milliseconds to wait=300) -> ()  [unwired: 1 out]
                              }
                            }
                          }
                        }
                      }
                      frame #3 {
                        n160 = local read "BAY 1"() -> (w399:u16)
                        n161 = local read "BAY 2"() -> (w398:u16)
                        n162 = local read "BAY 3"() -> (w397:u16)
                        n163 = local read "BAY 4"() -> (w396:u16)
                        n164 = local read "BAY 5"() -> (w395:u16)
                        n165 = local read "tube_id(in)"() -> (w406:enum16{".01", ".02", ".03", ".04"}[])
                        n166 = local read "Vr4"() -> (w409:dbl)
                        n167 = local read "tube_length(in)"() -> (w407:dbl[])
                        n168 = Build Array(w399, w398, w397, w396, w395) -> (w394:u16[])
                        n169 = local read "Vr3"() -> (w410:dbl)
                        n170 = local read "new_reactor_length"() -> (w404:bool[])
                        n171 = local read "Vr1"() -> (w412:dbl)
                        n172 = local read "Vr5"() -> (w408:dbl)
                        n173 = local read "Vr2"() -> (w411:dbl)
                        n174 = local read "new_reactor_volume"() -> (w402:bool[])
                        n175 = for {
                          N: 5 -> [_]
                          tunnel: w402 -> [w416] mode=indexing
                          tunnel: [w413] -> w400 mode=indexing
                          n176 = Select(t=1.0, s=w416, f=0.0) -> (s? t:f=w413:dbl)
                        }
                        n177 = for {
                          N: 5 -> [_]
                          tunnel: w404 -> [w420] mode=indexing
                          tunnel: [w417] -> w403 mode=indexing
                          n178 = Select(t=1.0, s=w420, f=0.0) -> (s? t:f=w417:dbl)
                        }
                        n179 = script code="tube_diameters = [.01,.02,.03,.04];\naddpath('C:\\Users\\Admin\\Dropbox (MIT)\\MoD Files\\MATLAB');\ncalculate_reactor_volumes;"("BayConfig"=w394, "Vr1"=w412, "Vr2"=w411, "Vr3"=w410, "Vr4"=w409, "Vr5"=w408, "tube_length"=w407, "tube_id"=w406, "new_len_react"=w403, "new_vol_react"=w400) -> ("Vr1"=w393:dbl, "Vr2"=w392:dbl, "Vr3"=w391:dbl, "Vr4"=w390:dbl, "Vr5"=w389:dbl)  [unwired: 1 in, 1 out]
                        n180 = local write "Vr1"(w393) -> ()
                        n181 = local write "Vr2"(w392) -> ()
                        n182 = local write "Vr3"(w391) -> ()
                        n183 = local write "Vr4"(w390) -> ()
                        n184 = local write "Vr5"(w389) -> ()
                      }
                      frame #4 {
                        n185 = local read "Setup Error"() -> (w423:bool)
                        n186 = case shown="True" w423 {
                          tunnel: [TRUE FALSE] -> w421
                          tunnel: ["" "Sytem setup has not been confirmed!"] -> w422
                          frame False {
                          }
                          frame True {
                            n187 = local read "Error Message"() -> (w428:string)
                            n188 = One Button Dialog(message=w428) -> ()  [unwired: 1 in, 1 out]
                          }
                        }
                        n189 = local write "System Confirm Not Clicked"(w422) -> ()
                        n190 = local write "Setup Confirm"(w421) -> ()
                      }
                    }
                  }
                }
              }
            }
            n191 = local read "Stop"() -> (w207:bool)
            n192 = Or(x=w208, y=w207) -> (x .or. y?=w206:bool)
            n193 = disable-structure shown="Disabled" {
              disable-tunnel: 400 -> [w214 _]
              frame Disabled {
                n194 = event shown="[1]" {
                  selector: _ -> [_ _]
                  dyn-events: _ -> [_ _]
                  timeout: w214 -> [_ _]
                  event Timeout {
                    n195 = event-data() -> ()  [unwired: 1 in, 3 out]
                  }
                  event #1 (no event record) {
                    n196 = event-data() -> ()  [unwired: 1 in, 6 out]
                    n197 = local read "Setup Confirm"() -> (w215:bool)
                    n198 = local read "Reaction Scheme Confirm"() -> (w216:bool)
                    n199 = Not(x=w215) -> (.not. x?=w218:bool)
                    n200 = And(x=w216, y=w218) -> (x .and. y?=w217:bool)
                    n201 = case shown="True" w217 {
                      frame False {
                      }
                      frame True {
                        w220 = u16 0 items=["                     Bypass", "                Hot Reactor", "                 Separator"] ("BAY 5")
                        w221 = u16 0 items=["                     Bypass", "                Hot Reactor", "                  Separator"] ("BAY 4")
                        w222 = u16 0 items=["                     Bypass", "                 Hot Reactor", "                  Separator"] ("BAY 3")
                        w223 = u16 0 items=["                     Bypass", "                Hot Reactor", "                  Separator"] ("BAY 2")
                        w224 = u16 0 items=["                 Bypass", "             Hot Reactor", "               Separator"] ("BAY 1")
                        n202 = local write "BAY 3"(w222) -> ()
                        n203 = local write "BAY 4"(w221) -> ()
                        n204 = local write "BAY 5"(w220) -> ()
                        n205 = local write "BAY 2"(w223) -> ()
                        n206 = local write "BAY 1"(w224) -> ()
                        n207 = local write "Synthesis Route Array"(string[][] [["3-Br-Pyridine _ Biphenyl", "K2CO3", "PhB(OH)2", "", "", ""]] ("Synthesis Route Array")) -> ()
                      }
                    }
                  }
                }
              }
              frame Enabled {
              }
            }
            n208 = disable-structure shown="Disabled" {
              disable-tunnel: 400 -> [w210 _]
              frame Disabled {
                n209 = event shown="[1]" {
                  selector: _ -> [_ _]
                  dyn-events: _ -> [_ _]
                  timeout: w210 -> [_ _]
                  event Timeout {
                    n210 = event-data() -> ()  [unwired: 1 in, 3 out]
                  }
                  event #1 (no event record) {
                    n211 = event-data() -> ()  [unwired: 1 in, 6 out]
                    n212 = call "File Dialog"("prompt"="Load previously saved xml file") -> ("selected path"=w212:path)  [unwired: 11 in, 3 out]
                    n213 = Path To String(path=w212) -> (string=w211:string)
                    n214 = script code="xmlDoc = xmlread(file_path);\nroot = xmlDoc.getDocumentElement();\nb = root.getChildNodes;\nrecipe = b.getElementsByTagName('Bay1').item(0);"("file_path"=w211) -> ()  [unwired: 1 in, 1 out]
                  }
                }
              }
              frame Enabled {
              }
            }
          }
        }
        frame #1 {
          n215 = local read "Stop"() -> (w430:bool)
          n216 = Not(x=w430) -> (.not. x?=w429:bool)
          n217 = case shown="True" w429 {
            tunnel: w431 -> [_ w434]
            frame False {
              "stop_button clicked" <- TRUE ("stop_button clicked")
            }
            frame True {
              # "Parameters Initilization"
              n218 = flat-sequence {
                tunnel: w434 -> [w436]
                tunnel: [w435] -> w433
                tunnel: w433 -> [w595]
                frame #0 {
                  # "Setup bays(RFID - verify)"
                  n219 = disable-structure shown="Disabled" {
                    frame Disabled {
                      n220 = local read "BAY 1"() -> ()  [unwired: 1 out]
                      n221 = local read "BAY 2"() -> ()  [unwired: 1 out]
                      n222 = local read "BAY 3"() -> ()  [unwired: 1 out]
                      n223 = local read "BAY 4"() -> ()  [unwired: 1 out]
                      n224 = local read "BAY 5"() -> ()  [unwired: 1 out]
                    }
                    frame Enabled {
                    }
                  }
                }
                frame #1 {
                  n225 = while {
                    tunnel: w436 -> [w439]
                    tunnel: [w438] -> w435
                    stop <- w442 stop-if-true
                    n226 = flat-sequence {
                      tunnel: [w456] -> w438
                      tunnel: w439 -> [w537]
                      tunnel: [w455] -> w437
                      frame #0 {
                        n227 = while {
                          stop <- w446 stop-if-true
                          n228 = event shown="[1] \"System Parameters Confirm Button\": Value Change" {
                            selector: _ -> [_ _]
                            dyn-events: _ -> [_ _]
                            timeout: u32 200 ("milliseconds to wait") -> [_ _]
                            tunnel: [FALSE TRUE] -> w444
                            event Timeout {
                              n229 = event-data() -> ()  [unwired: 1 in, 3 out]
                            }
                            event "System Parameters Confirm Button": Value Change {
                              n230 = event-data() -> ()  [unwired: 1 in, 5 out]
                              n231 = local write "System Parameters Confirm Button"(FALSE) -> ()
                            }
                          }
                          n232 = Wait (ms)(milliseconds to wait=u32 500) -> ()  [unwired: 1 out]
                          n233 = local read "Stop"() -> (w447:bool)
                          n234 = Or(x=w447, y=w444) -> (x .or. y?=w446:bool)
                        }
                      }
                      frame #1 {
                        w476 = 0 ("disabled index (col)")
                        w488 = 1 ("disabled index (col)")
                        # "Do while parameters have not been correctly entered"
                        n235 = local read "Bay Parameters"() -> (w475:T2)
                        n236 = local read "Synthesis Route Array"() -> (w489:string[][])
                        n237 = local read "Total Number of Experiments"() -> (w508:dbl)
                        n238 = Unbundle By Name(w475) -> ("Continue from previous optimization?"=w536:bool)
                        n239 = Unbundle By Name(w475) -> ("Excel File Name"=w538:string)
                        n240 = Unbundle By Name(w475) -> ("Matlab File"=w534:string)
                        n241 = Unbundle By Name(w475) -> ("Bay 1.Run at set flowrate"=w580:bool)
                        n242 = Unbundle By Name(w475) -> ("Bay 1.Pump 1 Flowrate"=w586:dbl)
                        n243 = Unbundle By Name(w475) -> ("Bay 1.Pump 2 Flowrate"=w585:dbl)
                        n244 = Unbundle By Name(w475) -> ("Bay 2.Run at set flowrate"=w578:bool)
                        n245 = Unbundle By Name(w475) -> ("Bay 2.Pump 3 Flowrate"=w584:dbl)
                        n246 = Unbundle By Name(w475) -> ("Bay 3.Pump 4 Flowrate"=w583:dbl)
                        n247 = Unbundle By Name(w475) -> ("Bay 3.Run at set flowrate"=w577:bool)
                        n248 = Unbundle By Name(w475) -> ("Bay 4.Run at set flowrate"=w574:bool)
                        n249 = Unbundle By Name(w475) -> ("Bay 4.Pump 5 Flowrate"=w582:dbl)
                        n250 = Unbundle By Name(w475) -> ("Bay 5.Pump 6 Flowrate"=w581:dbl)
                        n251 = Unbundle By Name(w475) -> ("Bay 5.Run at set flowrate"=w573:bool)
                        n252 = Index Array(array=w489, index (row)=3, index (col)=w488) -> (element=w482:string)
                        n253 = Index Array(array=w489, index (row)=2, index (col)=w488) -> (element=w480:string)
                        n254 = Index Array(array=w489, index (row)=1, index (col)=w488) -> (element=w478:string)
                        n255 = Index Array(array=w489, index (row)=0, index (col)=w488) -> (element=w491:string)
                        n256 = Index Array(array=w489, index (row)=4, index (col)=w488) -> (element=w484:string)
                        n257 = Index Array(array=w489, index (row)=5, index (col)=w488) -> (element=w486:string)
                        n258 = Build Array(w491, w478, w480, w482, w484, w486) -> (w492:string[])
                        n259 = Index Array(array=w489, index (row)=0 ("index"), index (col)=w476) -> (element=w514:string)
                        n260 = for {
                          tunnel: w492 -> [w588] mode=indexing
                          tunnel: [w587] -> w477 mode=indexing
                          n261 = script code="ctemp1 = str2num(c_temp);"("c_temp"=w588) -> ("ctemp1"=w587:dbl)  [unwired: 1 in, 1 out]
                        }
                        n262 = Boolean To (0,1)(Boolean=w578) -> (0, 1=w533:i16)
                        n263 = Boolean To (0,1)(Boolean=w574) -> (0, 1=w575:i16)
                        n264 = Boolean To (0,1)(Boolean=w577) -> (0, 1=w576:i16)
                        n265 = Boolean To (0,1)(Boolean=w536) -> (0, 1=w535:i16)
                        n266 = Boolean To (0,1)(Boolean=w580) -> (0, 1=w579:i16)
                        n267 = Boolean To (0,1)(Boolean=w573) -> (0, 1=w572:i16)
                        n268 = Index Array(array=w489, index (row)=1 ("index"), index (col)=w476) -> (element=w509:string)
                        n269 = Index Array(array=w489, index (row)=2 ("index"), index (col)=w476) -> (element=w510:string)
                        n270 = Unbundle By Name(w475) -> ("Bay 1.optimize_temp"=w571:bool)
                        n271 = Unbundle By Name(w475) -> ("Bay 1.optimize_tau"=w569:bool)
                        n272 = Unbundle By Name(w475) -> ("Bay 2.optimize_temp"=w567:bool)
                        n273 = Unbundle By Name(w475) -> ("Bay 2.optimize_tau"=w565:bool)
                        n274 = Unbundle By Name(w475) -> ("Bay 3.optimize_temp"=w563:bool)
                        n275 = Unbundle By Name(w475) -> ("Bay 3.optimize_tau"=w561:bool)
                        n276 = Unbundle By Name(w475) -> ("Bay 4.optimize_temp"=w559:bool)
                        n277 = Unbundle By Name(w475) -> ("Bay 4.optimize_tau"=w557:bool)
                        n278 = Index Array(array=w489, index (row)=3 ("index"), index (col)=w476) -> (element=w511:string)
                        n279 = Boolean To (0,1)(Boolean=w559) -> (0, 1=w558:i16)
                        n280 = Boolean To (0,1)(Boolean=w557) -> (0, 1=w556:i16)
                        n281 = Index Array(array=w489, index (row)=4 ("index"), index (col)=w476) -> (element=w512:string)
                        n282 = Boolean To (0,1)(Boolean=w561) -> (0, 1=w560:i16)
                        n283 = Boolean To (0,1)(Boolean=w567) -> (0, 1=w566:i16)
                        n284 = Boolean To (0,1)(Boolean=w571) -> (0, 1=w570:i16)
                        n285 = Boolean To (0,1)(Boolean=w565) -> (0, 1=w564:i16)
                        n286 = Boolean To (0,1)(Boolean=w569) -> (0, 1=w568:i16)
                        n287 = Boolean To (0,1)(Boolean=w563) -> (0, 1=w562:i16)
                        n288 = Unbundle By Name(w475) -> ("Bay 5.optimize_temp"=w555:bool)
                        n289 = Unbundle By Name(w475) -> ("Bay 5.optimize_tau"=w553:bool)
                        n290 = Index Array(array=w489, index (row)=5 ("index"), index (col)=w476) -> (element=w513:string)
                        n291 = Boolean To (0,1)(Boolean=w555) -> (0, 1=w554:i16)
                        n292 = Boolean To (0,1)(Boolean=w553) -> (0, 1=w552:i16)
                        n293 = Build Array(w570, w568, w566, w564, w562, w560, w558, w556, w554, w552) -> (w551:i16[])
                        n294 = Unbundle By Name(w475) -> ("Bay 1.Temperature Params"=w548:dbl[])
                        n295 = Unbundle By Name(w475) -> ("Bay 2.Temperature Params"=w547:dbl[])
                        n296 = Unbundle By Name(w475) -> ("Bay 2.Resisdence time params"=w542:dbl[])
                        n297 = Unbundle By Name(w475) -> ("Bay 3.Temperature Params"=w546:dbl[])
                        n298 = Unbundle By Name(w475) -> ("Bay 3.Resisdence time params"=w541:dbl[])
                        n299 = Unbundle By Name(w475) -> ("Bay 4.Temperature Params"=w545:dbl[])
                        n300 = Unbundle By Name(w475) -> ("Bay 4.Resisdence time params"=w540:dbl[])
                        n301 = Unbundle By Name(w475) -> ("Bay 5.Temperature Params"=w544:dbl[])
                        n302 = Unbundle By Name(w475) -> ("Bay 5.Resisdence time params"=w539:dbl[])
                        n303 = Unbundle By Name(w475) -> ("Bay 1.pump params 2"=w507:dbl[])
                        n304 = Unbundle By Name(w475) -> ("Bay 1.pump params 1"=w543:dbl[])
                        n305 = Unbundle By Name(w475) -> ("Bay 1.Run at set temperature"=w498:bool)
                        n306 = Unbundle By Name(w475) -> ("Bay 2.Run at set temperature"=w496:bool)
                        n307 = Unbundle By Name(w475) -> ("Bay 3.Run at set temperature"=w495:bool)
                        n308 = Unbundle By Name(w475) -> ("Bay 4.Run at set temperature"=w494:bool)
                        n309 = Unbundle By Name(w475) -> ("Bay 5.Run at set temperature"=w493:bool)
                        n310 = Unbundle By Name(w475) -> ("Bay 3.Temperature"=w504:dbl)
                        n311 = Unbundle By Name(w475) -> ("Bay 1.Temperature"=w506:dbl)
                        n312 = Unbundle By Name(w475) -> ("Bay 2.Temperature"=w505:dbl)
                        n313 = Unbundle By Name(w475) -> ("Bay 4.Temperature"=w503:dbl)
                        n314 = Unbundle By Name(w475) -> ("Bay 5.Temperature"=w502:dbl)
                        n315 = Unbundle By Name(w475) -> ("Bay 3.pump_num_ratio"=w527:dbl)
                        n316 = Unbundle By Name(w475) -> ("Bay 4.pump_num_ratio"=w524:dbl)
                        n317 = Unbundle By Name(w475) -> ("Bay 5.pump_num_ratio"=w521:dbl)
                        n318 = Unbundle By Name(w475) -> ("Bay 2.pump_num_ratio"=w530:dbl)
                        n319 = Unbundle By Name(w475) -> ("Bay 4.pump_at_ratio"=w526:bool)
                        n320 = Boolean To (0,1)(Boolean=w526) -> (0, 1=w525:i16)
                        n321 = Unbundle By Name(w475) -> ("Bay 3.pump_at_ratio"=w529:bool)
                        n322 = Boolean To (0,1)(Boolean=w529) -> (0, 1=w528:i16)
                        n323 = Unbundle By Name(w475) -> ("Bay 5.pump_at_ratio"=w523:bool)
                        n324 = Boolean To (0,1)(Boolean=w523) -> (0, 1=w522:i16)
                        n325 = Unbundle By Name(w475) -> ("Bay 2.pump_at_ratio"=w532:bool)
                        n326 = Boolean To (0,1)(Boolean=w532) -> (0, 1=w531:i16)
                        n327 = Build Array(w506, w505, w504, w503, w502) -> (w501:dbl[])
                        n328 = Build Array(w498, w496, w495, w494, w493) -> (w497:bool[])
                        n329 = local read "Syringe_pump?"() -> (w454:bool)
                        n330 = for {
                          N: 5 -> [_]
                          tunnel: w497 -> [w592] mode=indexing
                          tunnel: [w591] -> w499 mode=indexing
                          n331 = Select(t=1.0, s=w592, f=0.0) -> (s? t:f=w591:dbl)
                        }
                        n332 = Unbundle By Name(w475) -> ("Internal Standard?"=w466:bool)
                        n333 = Unbundle By Name(w475) -> ("increas_decrease_hplc_peak"=w467:bool)
                        n334 = Unbundle By Name(w475) -> ("Hplc Wait time(min)"=w459:dbl)
                        n335 = Unbundle By Name(w475) -> ("Total Number of Experiments 2"=w458:dbl)
                        n336 = Unbundle By Name(w475) -> ("hplc_start"=w463:dbl)
                        n337 = Unbundle By Name(w475) -> ("ISTD start"=w461:dbl)
                        n338 = Unbundle By Name(w475) -> ("hplc_end"=w462:dbl)
                        n339 = Unbundle By Name(w475) -> ("throughput_yield"=w468:bool)
                        n340 = Unbundle By Name(w475) -> ("ISTD end"=w460:dbl)
                        n341 = Select(t=1.0, s=w454, f=0.0) -> (s? t:f=w453:dbl)
                        n342 = Select(t=1.0, s=w467, f=0.0) -> (s? t:f=w465:dbl)
                        n343 = Select(t=1.0, s=w466, f=0.0) -> (s? t:f=w464:dbl)
                        n344 = Select(t=0.0, s=w468, f=1.0) -> (s? t:f=w457:dbl)
                        n345 = script code="system_error = 0;\nnumPeaks = 1;\nstart_phase_time = 1;\nis_redo_exp = 0;\nFvalues = [];\nHPLC_Area = [];\n\nT1_span = [1 1]; T2_span = [1 1]; T3_span = [1 1]; T4_span = [1 1]; T5_span = [1 1];\nT_span = [T1_span;T2_span;T3_span;T4_span;T5_span];\n p1_span =  [1 1]; p2_span =  [1 1]; p3_span =  [1 1]; p4_span =  [1 1]; p5_span =  [1 1];  p6_span =  [1 1];\nOpt_params = [0 0 0 0 0 0 0 0 0 0 0];\nT_params = [T1_params;T2_params;T3_params;T4_params;T5_params];\npump_params = [pump1_params;pump2_params;pump3_params;pump4_params;pump5_params;pump6_params];\nopt_ctr = 0;ncall = 100;record_data = true;\nT1_SP = 23; T2_SP = 23; T3_SP = 23; T4_SP = 23; T5_SP = 23;\nT_span = [T1_span;T2_span;T3_span;T4_span;T5_span];\np_span = [p1_span;p2_span;p3_span;p4_span;p5_span;p6_span];\nno_errors = 1;\nP1 = 0; P2 =0; P3 = 0; P4 = 0; P5 = 0; P6 = 0;\nP = [P1, P2, P3,P4, P5, P6];\nis_first_set_of_exp = true;\nerror_message = 'System has no errors to report';\n%addpath(genpath('C:\\Users\\HPLC\\Dropbox (MIT)\\MoD Files\\MATLAB'))\naddpath(genpath('C:\\Users\\Admin\\Dropbox (MIT)\\MoD Files\\MATLAB'))\nallMSData = [];allHPLCData = [];allHPLCFile = [];\nBay_ratio = [0,Bay2_ratio,Bay3_ratio,Bay4_ratio,Bay5_ratio];\nBay_pump_ratio = [1, Bay2_pump_ratio, Bay3_pump_ratio, Bay4_pump_ratio, Bay5_pump_ratio];\nP_setrate = [P1_setrate, P2_setrate, P3_setrate, P4_setrate, P5_setrate, P6_setrate];\nuse_flowrate = [use_flowrate1, use_flowrate2,use_flowrate3, use_flowrate4, use_flowrate5];\npump_chem_name= []\nCurrExp = 1;\n% ****************************************************************************************************\n%Setup optimization\n   setup_optimization_params;\n   initialize_opt = 0;\n   nstop0 = 0;\n%*****************************************************************************************************\n% Setup excel and xml file writing\npath(path, pa);\nnumMSSig = 1;\nsetup_excel_output;\n%***************************************************************************************************\nredo = false;\nncall = ncall_in;"("use_flowrate1"=w579, "P1_setrate"=w586, "P2_setrate"=w585, "P3_setrate"=w584, "P4_setrate"=w583, "P5_setrate"=w582, "P6_setrate"=w581, "use_flowrate2"=w533, "use_flowrate3"=w576, "use_flowrate4"=w575, "use_flowrate5"=w572, "Optimize_params"=w551, "T1_params"=w548, "T2_params"=w547, "T3_params"=w546, "T4_params"=w545, "T5_params"=w544, "pump1_params"=w543, "pump3_params"=w542, "pump4_params"=w541, "pump5_params"=w540, "pump6_params"=w539, "xl_file"=w538, "pa"=w537, "Continue"=w535, "matlabsavefile"=w534, "Bay2_ratio"=w531, "Bay2_pump_ratio"=w530, "Bay3_ratio"=w528, "Bay3_pump_ratio"=w527, "Bay4_ratio"=w525, "Bay4_pump_ratio"=w524, "Bay5_ratio"=w522, "Bay5_pump_ratio"=w521, "pump1_chem"=w514, "pump6_chem"=w513, "pump5_chem"=w512, "pump4_chem"=w511, "pump3_chem"=w510, "pump2_chem"=w509, "Pump_concen"=w477, "ncall_in"=w508, "pump2_params"=w507, "T_SP"=w501, "Run_at_T_SP"=w499, "dcr_hplc_peak"=w465, "use_internal_std"=w464, "hplc_peak_start"=w463, "hplc_peak_end"=w462, "ISTD_start"=w461, "ISTD_end"=w460, "hplc_wait_time"=w459, "tot_num_exp"=w458, "throughput_yield"=w457, "syringe_pump"=w453) -> ("no_errors"=w550:dbl, "error_message"=w549:string)  [unwired: 1 in, 1 out]
                        n346 = Not Equal To 0?(x=w550) -> (x != 0?=w455:bool)
                        n347 = Not(x=w455) -> (.not. x?=w456:bool)
                        n348 = case shown="False" w456 {
                          tunnel: w549 -> [_ w594]
                          frame False {
                            n349 = local write "Setup Confirm 2"(TRUE ("Setup Confirm 2")) -> ()
                          }
                          frame True {
                            n350 = One Button Dialog(message=w594) -> ()  [unwired: 1 in, 1 out]
                          }
                        }
                      }
                    }
                    n351 = local read "Stop"() -> (w441:bool)
                    n352 = Or(x=w437, y=w441) -> (x .or. y?=w442:bool)
                    n353 = Wait (ms)(milliseconds to wait=u32 500) -> ()  [unwired: 1 out]
                  }
                }
                frame #2 {
                  n354 = local write "System Error"(w595) -> ()
                }
              }
            }
          }
        }
        frame #2 {
          # "Run Initial diagnostics"
        }
        frame #3 {
          # "Run System"
          n355 = while {
            tunnel: w596 -> [w1307]
            stop <- w1311 stop-if-true
            n356 = local read "running?"() -> (w1306:bool)
            n357 = local read "Temperature Control 1"() -> (w1308:bool)
            n358 = And(x=w1306, y=w1308) -> (x .and. y?=w1309:bool)
            n359 = case shown="True" w1309 {
              tunnel: w1307 -> [_ w1313]
              frame False {
                n360 = local write "Temp SS? 1"(TRUE ("Temp SS? 1")) -> ()
              }
              frame True {
                # "Bay 1 Temperature Controller"
                n361 = local read "Temperature SP 1"() -> (w1314:dbl)
                n362 = local read "Temperature 1"() -> (w1318:dbl)
                n363 = local read "SSR Duration 1"() -> (w1333:dbl)
                n364 = call-poly <vilib>:"PID Online Autotuning.vi"("setpoint"=w1314, "manipulated variable"=w1333, "autotuning parameters"=T9 {"type of controller"=enum."PID", "relay cycles"=3, "relay amplitude"=1.0, "control specifications"=enum."Normal", "PV noise level"=0.1} ("Autotuning Parameters R1"), "process variable"=w1318, "PID gains in"=T8 {"Proportional gain Kc"=0.38538, "Integral time Ti (sec)"=0.524375, "Derivative time Ti (sec)"=0.12585} ("PID gains 2")) -> ("setpoint out"=w1339:dbl, "process variable out"=w1338:dbl, "PID gains out"=w1335:T17)  [unwired: 6 in, 2 out]
                n365 = call <vilib>:"PID Autotuning (Temperature).vi"("desired temperature"=w1339, "measured temperature"=w1338, "plant parameters in"=w1335, "output range"=cluster{"output high":dbl, "output low":dbl} {"output high"=3.0, "output low"=-1.0} ("Output range")) -> ("output"=w1331:dbl)  [unwired: 12 in, 3 out]
                n366 = local write "SSR Duration 1"(w1331) -> ()
                n367 = Subtract(x=w1314, y=w1318) -> (x-y=w1325:dbl)
                n368 = Absolute Value(x=w1325) -> (abs(x)=w1328:dbl)
                n369 = Multiply(x=1000.0, y=w1331) -> (x*y=w1329:dbl)
                n370 = Greater Than 0?(x=w1329) -> (x > 0?=w1323:bool)
                n371 = Less Or Equal?(x=w1328, y=1.2) -> (x <= y?=w1326:bool)
                n372 = Greater?(x=w1314, y=w1318) -> (0:w1324:bool)
                n373 = And(x=w1323, y=w1324) -> (x .and. y?=w1321:bool)
                n374 = local write "Temp SS? 1"(w1326) -> ()
                n375 = Subtract(x=w1318, y=10.0) -> (x-y=w1319:dbl)
                n376 = Less?(x=w1319, y=w1314) -> (x < y?=w1322:bool)
                n377 = And(x=w1322, y=w1321) -> (x .and. y?=w1320:bool)
                n378 = case shown="True" w1320 {
                  tunnel: [errorcluster {"status"=FALSE, "code"=0, "source"=""} ("error out") w1349] -> _
                  tunnel: 2 -> [_ w1346]
                  tunnel: w1329 -> [w1343 w1347]
                  tunnel: [0.0 w1351] -> w1316
                  tunnel: w1314 -> [_ w1350]
                  tunnel: w1313 -> [_ w1348]
                  frame False {
                    n379 = Absolute Value(x=w1343) -> (abs(x)=w1344:dbl)
                    n380 = Wait (ms)(milliseconds to wait=w1344) -> ()  [unwired: 1 out]
                  }
                  frame True {
                    n381 = call "TurnOnRelayArduino.vi"("channel"=w1346, "duration"=w1347, "LINX Resource"=w1348) -> ("error out"=w1349:errorcluster)  [unwired: 7 in, 1 out]
                    n382 = script code="tempdiff1= SP1 - T1;\nif tempdiff1 > 10\n  if slope1 < .01\n     temp_check1 = temp_check1 + 1;\n  else\n      temp_check1 =0;\n  end\nend\n\nif temp_check1 > 9\n  temp_error1 = 1\nend"("SP1"=w1350) -> ("temp_error1"=w1351:dbl)  [unwired: 1 in, 1 out]
                  }
                }
                n383 = Not Equal To 0?(x=w1316) -> (x != 0?=w1315:bool)
                n384 = case shown="True" w1315 {
                  frame False {
                  }
                  frame True {
                    n385 = local write "Error Message"("Bay 1 Temperature Heating Error") -> ()
                  }
                }
                n386 = case shown="True" w1315 {
                  tunnel: w1315 -> [_ w1341]
                  frame False {
                  }
                  frame True {
                    n387 = local write "System Error"(w1341) -> ()
                    n388 = local write "Stop"(w1341) -> ()
                  }
                }
              }
            }
            n389 = Wait (ms)(milliseconds to wait=u32 400) -> ()  [unwired: 1 out]
            n390 = local read "Stop"() -> (w1311:bool)
          }
          n391 = local read "Bay Parameters"() -> (w600:T2)
          n392 = while {
            tunnel: w596 -> [w1261]
            stop <- w1265 stop-if-true
            n393 = local read "running?"() -> (w1260:bool)
            n394 = local read "Temperature Control 2"() -> (w1262:bool)
            n395 = And(x=w1260, y=w1262) -> (x .and. y?=w1263:bool)
            n396 = case shown="True" w1263 {
              tunnel: w1261 -> [_ w1267]
              frame False {
                n397 = local write "Temp SS? 2"(TRUE ("Temp SS? 2")) -> ()
              }
              frame True {
                # "Bay 2 Temperature Controller"
                n398 = local read "Temperature SP 2"() -> (w1269:dbl)
                n399 = local read "Temperature 2"() -> (w1272:dbl)
                n400 = local read "SSR Duration 2"() -> (w1290:dbl)
                n401 = call-poly <vilib>:"PID Online Autotuning.vi"("setpoint"=w1269, "manipulated variable"=w1290, "autotuning parameters"=T9 {"type of controller"=enum."PID", "relay cycles"=3, "relay amplitude"=1.0, "control specifications"=enum."Normal", "PV noise level"=0.1} ("Autotuning Parameters R1"), "process variable"=w1272, "PID gains in"=T8 {"Proportional gain Kc"=0.38538, "Integral time Ti (sec)"=0.524375, "Derivative time Ti (sec)"=0.12585} ("PID gains 2")) -> ("setpoint out"=w1288:dbl, "process variable out"=w1287:dbl, "PID gains out"=w1293:T17)  [unwired: 6 in, 2 out]
                n402 = call <vilib>:"PID Autotuning (Temperature).vi"("desired temperature"=w1288, "measured temperature"=w1287, "plant parameters in"=w1293, "output range"=cluster{"output high":dbl, "output low":dbl} {"output high"=3.0, "output low"=-1.0} ("Output range")) -> ("output"=w1283:dbl)  [unwired: 12 in, 3 out]
                n403 = local write "SSR Duration 2"(w1283) -> ()
                n404 = Greater?(x=w1269, y=w1272) -> (0:w1278:bool)
                n405 = Multiply(x=1000.0, y=w1283) -> (x*y=w1285:dbl)
                n406 = Greater Than 0?(x=w1285) -> (x > 0?=w1277:bool)
                n407 = And(x=w1277, y=w1278) -> (x .and. y?=w1275:bool)
                n408 = Subtract(x=w1269, y=w1272) -> (x-y=w1280:dbl)
                n409 = Absolute Value(x=w1280) -> (abs(x)=w1282:dbl)
                n410 = Subtract(x=w1272, y=10.0) -> (x-y=w1274:dbl)
                n411 = Less Or Equal?(x=w1282, y=1.2) -> (x <= y?=w1279:bool)
                n412 = local write "Temp SS? 2"(w1279) -> ()
                n413 = Less?(x=w1274, y=w1269) -> (x < y?=w1276:bool)
                n414 = And(x=w1276, y=w1275) -> (x .and. y?=w1271:bool)
                n415 = case shown="True" w1271 {
                  tunnel: [errorcluster {"status"=FALSE, "code"=0, "source"=""} ("error out") w1303] -> _
                  tunnel: 3 -> [_ w1300]
                  tunnel: w1285 -> [w1297 w1301]
                  tunnel: [0.0 w1305] -> w1270
                  tunnel: w1269 -> [_ w1304]
                  tunnel: w1267 -> [_ w1302]
                  frame False {
                    n416 = Absolute Value(x=w1297) -> (abs(x)=w1298:dbl)
                    n417 = Wait (ms)(milliseconds to wait=w1298) -> ()  [unwired: 1 out]
                  }
                  frame True {
                    n418 = call "TurnOnRelayArduino.vi"("channel"=w1300, "duration"=w1301, "LINX Resource"=w1302) -> ("error out"=w1303:errorcluster)  [unwired: 7 in, 1 out]
                    n419 = script code="tempdiff2= SP2 - T2;\nif tempdiff2 > 10\n  if slope2 < .01\n     temp_check2 = temp_check2 + 1;\n  else\n      temp_check2 =0;\n  end\nend\n\nif temp_check2 > 9\n  temp_error2 = 1\nend"("SP2"=w1304) -> ("temp_error2"=w1305:dbl)  [unwired: 1 in, 1 out]
                  }
                }
                n420 = Not Equal To 0?(x=w1270) -> (x != 0?=w1268:bool)
                n421 = case shown="True" w1268 {
                  frame False {
                  }
                  frame True {
                    n422 = local write "Error Message"("Bay 2 Temperature Heating Error") -> ()
                  }
                }
                n423 = case shown="True" w1268 {
                  tunnel: w1268 -> [_ w1295]
                  frame False {
                  }
                  frame True {
                    n424 = local write "Stop"(w1295) -> ()
                    n425 = local write "System Error"(w1295) -> ()
                  }
                }
              }
            }
            n426 = local read "Stop"() -> (w1265:bool)
            n427 = Wait (ms)(milliseconds to wait=u32 400) -> ()  [unwired: 1 out]
          }
          n428 = local read "Stop"() -> (w597:bool)
          n429 = Not(x=w597) -> (.not. x?=w599:bool)
          n430 = case shown="True" w599 {
            tunnel: w600 -> [_ w605]
            tunnel: w598 -> [_ w604]
            tunnel: w596 -> [_ w603]
            frame False {
            }
            frame True {
              n431 = while {
                tunnel: w605 -> [w619]
                tunnel: w604 -> [w611]
                tunnel: w603 -> [w606]
                i -> [w618]
                stop <- w612 stop-if-true
                n432 = local read "running?"() -> (w607:bool)
                n433 = Wait (ms)(milliseconds to wait=u32 1000) -> ()  [unwired: 1 out]
                n434 = Increment(x=w618) -> (x+1=w608:i32)
                n435 = case shown="True" w607 {
                  tunnel: w618 -> [w624 _]
                  tunnel: w619 -> [_ _]
                  tunnel: [w626 w630] -> w609
                  tunnel: [0.0 w631] -> w614
                  tunnel: w611 -> [_ w629]
                  tunnel: w606 -> [_ w627]
                  frame False {
                    # "STANDBY MODE"
                    n436 = Add(x=w624, y=2.0) -> (x+y=w626:dbl)
                  }
                  frame True {
                    n437 = flat-sequence {
                      tunnel: w629 -> [w633]
                      tunnel: [w633] -> w628
                      tunnel: [w643] -> w631
                      tunnel: [200.0] -> w630
                      tunnel: w628 -> [w641]
                      tunnel: w627 -> [w635]
                      frame #0 {
                        n438 = local write "stop_xl_write"(FALSE ("stop_xl_write")) -> ()
                      }
                      frame #1 {
                        # "Increase flowrate of dilution stream"
                        # "Wait mixed stream reaches SL"
                        # "SNOBFIT"
                        # "Optimize"
                        # "Run Experimental Conditions"
                        # "Optimize/Synthesize"
                        n439 = local read "Syringe_pump?"() -> (w634:bool)
                        n440 = local read "Stop"() -> (w638:bool)
                        n441 = Not(x=w638) -> (.not. x?=w637:bool)
                        n442 = case shown="True" w637 {
                          tunnel: [1.0 w666] -> w646
                          tunnel: [w654 w665] -> w640
                          tunnel: [0.0 w664] -> w639
                          tunnel: [w654 w663] -> w636
                          tunnel: w634 -> [_ w660]
                          frame False {
                            w654 = dbl[] []
                          }
                          frame True {
                            n443 = Select(t=1.0, s=w660, f=0.0) -> (s? t:f=w659:dbl)
                            n444 = script code="optimization_main_loop"("syringe_pump"=w659) -> ("Conditions_Array"=w665:dbl[], "opt_ctr"=w666:dbl, "P_tot"=w664:dbl, "tau_array"=w663:dbl[], "experiment_history"=w661:dbl[][])  [unwired: 1 in, 1 out]
                            n445 = call-poly <vilib>:"Array To Matrix.vi"("Real 2D Array"=w661) -> ("Real Matrix"=w662:T18)
                            n446 = local write "experiment history"(w662) -> ()
                          }
                        }
                        "P_tot" <- w639
                        n447 = local read "COMM Port :: Milligat Pumps"() -> (w647:refnum<visa-resource-name>)
                        n448 = Equal?(x=w646, y=1.0) -> (x = y?=w644:bool)
                        n449 = flat-sequence {
                          tunnel: w640 -> [w1105]
                          tunnel: w636 -> [w1099]
                          frame #0 {
                            # "Start recording data"
                            n450 = Index Array(array=w1105, index=5) -> (element=w1117:dbl)
                            n451 = Index Array(array=w1105, index=0) -> (element=w1112:dbl)
                            n452 = Index Array(array=w1105, index=1) -> (element=w1113:dbl)
                            n453 = Index Array(array=w1105, index=2) -> (element=w1115:dbl)
                            n454 = Index Array(array=w1105, index=3) -> (element=w1114:dbl)
                            n455 = Index Array(array=w1105, index=4) -> (element=w1116:dbl)
                            n456 = local write "Pump setpoint(ul/min) 2"(w1113) -> ()
                            n457 = local write "Pump setpoint(ul/min) 4"(w1115) -> ()
                            n458 = local write "Pump setpoint(ul/min) 5"(w1116) -> ()
                            n459 = local write "Pump setpoint(ul/min) 3"(w1114) -> ()
                            n460 = local write "Pump setpoint(ul/min) 6"(w1117) -> ()
                            n461 = local write "Pump setpoint(ul/min) 1"(w1112) -> ()
                            n462 = Index Array(array=w1099, index=0) -> (element=w1104:dbl)
                            n463 = Index Array(array=w1099, index=4) -> (element=w1103:dbl)
                            n464 = Index Array(array=w1099, index=3) -> (element=w1102:dbl)
                            n465 = Index Array(array=w1099, index=2) -> (element=w1101:dbl)
                            n466 = Index Array(array=w1099, index=1) -> (element=w1100:dbl)
                            n467 = local write "tau 2"(w1100) -> ()
                            n468 = local write "tau 3"(w1101) -> ()
                            n469 = local write "tau 4"(w1102) -> ()
                            n470 = local write "tau 5"(w1103) -> ()
                            n471 = local write "tau 1"(w1104) -> ()
                          }
                        }
                        n472 = flat-sequence {
                          tunnel: w647 -> [w670]
                          tunnel: w640 -> [w669]
                          tunnel: w644 -> [w668]
                          tunnel: [w668] -> w653
                          tunnel: w641 -> [w667]
                          tunnel: w653 -> [w836]
                          tunnel: [w836] -> w652
                          tunnel: w652 -> [w856]
                          tunnel: [w854] -> w651
                          tunnel: w640 -> [w880]
                          tunnel: w651 -> [w879]
                          tunnel: w635 -> [w878]
                          tunnel: [w1034] -> w650
                          tunnel: w650 -> [w1047]
                          tunnel: [w1047] -> w649
                          tunnel: w649 -> [w1055]
                          tunnel: [w1055] -> w648
                          tunnel: [w1093] -> w643
                          tunnel: w648 -> [w1093]
                          frame #0 {
                            # "Setup pump flowrates and temperature setpoints"
                            n473 = stacked-sequence {
                              tunnel: w670 -> [w696 _ _ _ _]
                              tunnel: w670 -> [_ w742 _ _ _]
                              tunnel: w670 -> [_ _ w770 _ _]
                              tunnel: w670 -> [_ _ _ w798 _]
                              tunnel: w670 -> [_ _ _ _ w826]
                              tunnel: w669 -> [w693 w740 w768 w796 w823]
                              tunnel: w668 -> [w685 w735 w763 w791 w819]
                              tunnel: w667 -> [w683 _ _ _ _]
                              frame #0 {
                                # "Bay 1"
                                n474 = local read "Syringe_pump?"() -> (w684:bool)
                                n475 = Index Array(array=w693, index=0) -> (element=w691:dbl)
                                n476 = local read "BAY 1"() -> (w678:u16)
                                n477 = Index Array(array=w693, index=1) -> (element=w690:dbl)
                                n478 = Index Array(array=w693, index=6) -> (element=w673:dbl)
                                n479 = script code="MATLAB script"("T1_SP"=w673) -> ()  [unwired: 1 in, 1 out]
                                n480 = Less Or Equal?(x=w678, y=u16 4) -> (x <= y?=w680:bool)
                                n481 = Greater Or Equal?(x=w678, y=u16 1) -> (x >= y?=w681:bool)
                                n482 = Not Equal?(x=23.0, y=w673) -> (x != y?=w674:bool)
                                n483 = And(x=w681, y=w680) -> (x .and. y?=w682:bool)
                                n484 = Greater Than 0?(x=w691) -> (x > 0?=w689:bool)
                                n485 = And(x=w689, y=w685) -> (x .and. y?=w688:bool)
                                n486 = Greater Than 0?(x=w690) -> (x > 0?=w687:bool)
                                n487 = Wait (ms)(milliseconds to wait=u32 300) -> ()  [unwired: 1 out]
                                n488 = And(x=w687, y=w685) -> (x .and. y?=w686:bool)
                                n489 = And(x=w682, y=w685) -> (x .and. y?=w672:bool)
                                n490 = And(x=w674, y=w672) -> (x .and. y?=w671:bool)
                                n491 = case shown="False" w684 {
                                tunnel: w696 -> [w699 _]
                                tunnel: w690 -> [w698 w706]
                                tunnel: w686 -> [w697 w707]
                                tunnel: w683 -> [_ w705]
                                frame False {
                                n492 = case shown="False" w697 {
                                tunnel: w699 -> [w701 w702]
                                tunnel: w698 -> [_ w703]
                                frame False {
                                n493 = call "PumpStop.vi"("Pump Address"="g", "Pump COMM Port"=w701) -> ()  [unwired: 9 in, 1 out]
                                }
                                frame True {
                                n494 = call "PumpDispense.vi"("Flowrate(ul/min)"=w703, "Pump Address"="g", "Pump COMM Port"=w702) -> ()  [unwired: 7 in, 2 out]
                                }
                                }
                                }
                                frame True {
                                n495 = case shown="True" w707 {
                                tunnel: w706 -> [_ w710]
                                tunnel: w705 -> [w709 w713]
                                frame False {
                                n496 = call <instrlib>:"Stop.vi"("VISA IN"=w709, "Pump Address"=i8 0) -> ()  [unwired: 7 in, 7 out]
                                }
                                frame True {
                                w711 = u16 0 items=["uL/min", "uL/hr", "mL/min", "mL/hr"] ("Units")
                                w712 = i8 0 ("Pump Address")
                                n497 = call <instrlib>:"WriteSP.vi"("VISA IN"=w713, "Pump Address"=w712, "SP"=w710, "Units"=w711) -> ("Error Out"=w714:errorcluster)  [unwired: 5 in, 6 out]
                                n498 = call <instrlib>:"Start.vi"("VISA IN"=w713, "Pump Address"=w712, "Error In (no error)"=w714) -> ()  [unwired: 6 in, 7 out]
                                }
                                }
                                }
                                }
                                n499 = case shown="False" w688 {
                                tunnel: w696 -> [w718 w720]
                                tunnel: w691 -> [_ w721]
                                frame False {
                                n500 = call "PumpStop.vi"("Pump Address"="f", "Pump COMM Port"=w718) -> ()  [unwired: 9 in, 1 out]
                                }
                                frame True {
                                n501 = call "PumpDispense.vi"("Flowrate(ul/min)"=w721, "Pump Address"="f", "Pump COMM Port"=w720) -> ()  [unwired: 7 in, 2 out]
                                }
                                }
                                n502 = case shown="True" w671 {
                                tunnel: w673 -> [_ w717]
                                frame False {
                                n503 = local write "Temperature Control 1"(FALSE) -> ()
                                }
                                frame True {
                                n504 = local write "Temperature SP 1"(w717) -> ()
                                n505 = local write "Temperature Control 1"(TRUE ("Temperature Control 1")) -> ()
                                }
                                }
                              }
                              frame #1 {
                                # "Bay 2"
                                n506 = local read "BAY 2"() -> (w731:u16)
                                n507 = Index Array(array=w740, index=2) -> (element=w738:dbl)
                                n508 = Index Array(array=w740, index=7) -> (element=w725:dbl)
                                n509 = script code="MATLAB script"("T2_SP"=w725) -> ()  [unwired: 1 in, 1 out]
                                n510 = Greater Than 0?(x=w738) -> (x > 0?=w737:bool)
                                n511 = And(x=w737, y=w735) -> (x .and. y?=w736:bool)
                                n512 = Not Equal?(x=23.0, y=w725) -> (x != y?=w726:bool)
                                n513 = Greater Or Equal?(x=w731, y=u16 1) -> (x >= y?=w729:bool)
                                n514 = Less Or Equal?(x=w731, y=u16 4) -> (x <= y?=w734:bool)
                                n515 = And(x=w729, y=w734) -> (x .and. y?=w733:bool)
                                n516 = And(x=w733, y=w735) -> (x .and. y?=w724:bool)
                                n517 = And(x=w726, y=w724) -> (x .and. y?=w723:bool)
                                n518 = case shown="True" w723 {
                                tunnel: w725 -> [_ w749]
                                frame False {
                                n519 = local write "Temperature Control 2"(FALSE) -> ()
                                }
                                frame True {
                                n520 = local write "Temperature Control 2"(TRUE ("Temperature Control 2")) -> ()
                                n521 = local write "Temperature SP 2"(w749) -> ()
                                }
                                }
                                n522 = case shown="False" w736 {
                                tunnel: w738 -> [_ w745]
                                tunnel: w742 -> [w743 w746]
                                frame False {
                                n523 = call "PumpStop.vi"("Pump Address"="i", "Pump COMM Port"=w743) -> ()  [unwired: 9 in, 1 out]
                                }
                                frame True {
                                n524 = call "PumpDispense.vi"("Flowrate(ul/min)"=w745, "Pump Address"="i", "Pump COMM Port"=w746) -> ()  [unwired: 7 in, 2 out]
                                }
                                }
                                n525 = Wait (ms)(milliseconds to wait=u32 300) -> ()  [unwired: 1 out]
                              }
                              frame #2 {
                                # "Bay 3"
                                n526 = local read "BAY 3"() -> (w758:u16)
                                n527 = Index Array(array=w768, index=3) -> (element=w766:dbl)
                                n528 = Not Equal To 0?(x=w766) -> (x != 0?=w765:bool)
                                n529 = Index Array(array=w768, index=8) -> (element=w751:dbl)
                                n530 = script code="MATLAB script"("T3_SP"=w751) -> ()  [unwired: 1 in, 1 out]
                                n531 = Less Or Equal?(x=w758, y=u16 4) -> (x <= y?=w762:bool)
                                n532 = Greater Or Equal?(x=w758, y=u16 1) -> (x >= y?=w759:bool)
                                n533 = And(x=w759, y=w762) -> (x .and. y?=w757:bool)
                                n534 = And(x=w757, y=w763) -> (x .and. y?=w753:bool)
                                n535 = And(x=w765, y=w763) -> (x .and. y?=w764:bool)
                                n536 = Not Equal?(x=23.0, y=w751) -> (x != y?=w754:bool)
                                n537 = And(x=w754, y=w753) -> (x .and. y?=w752:bool)
                                n538 = case shown="False" w764 {
                                tunnel: w766 -> [_ w773]
                                tunnel: w770 -> [w771 w774]
                                frame False {
                                n539 = call "PumpStop.vi"("Pump Address"="e", "Pump COMM Port"=w771) -> ()  [unwired: 9 in, 1 out]
                                }
                                frame True {
                                n540 = call "PumpDispense.vi"("Flowrate(ul/min)"=w773, "Pump Address"="e", "Pump COMM Port"=w774) -> ()  [unwired: 7 in, 2 out]
                                }
                                }
                                n541 = case shown="False" w752 {
                                tunnel: w751 -> [_ w777]
                                frame False {
                                n542 = local write "Temperature Control 3"(FALSE) -> ()
                                }
                                frame True {
                                n543 = local write "Temperature Control 3"(TRUE ("Temperature Control 3")) -> ()
                                n544 = local write "Temperature SP 3"(w777) -> ()
                                }
                                }
                                n545 = Wait (ms)(milliseconds to wait=u32 300) -> ()  [unwired: 1 out]
                              }
                              frame #3 {
                                # "Bay 4"
                                n546 = Index Array(array=w796, index=9) -> (element=w779:dbl)
                                n547 = script code="MATLAB script"("T4_SP"=w779) -> ()  [unwired: 1 in, 1 out]
                                n548 = Index Array(array=w796, index=4) -> (element=w794:dbl)
                                n549 = Not Equal To 0?(x=w794) -> (x != 0?=w793:bool)
                                n550 = local read "BAY 4"() -> (w785:u16)
                                n551 = And(x=w793, y=w791) -> (x .and. y?=w792:bool)
                                n552 = Less Or Equal?(x=w785, y=u16 4) -> (x <= y?=w790:bool)
                                n553 = Greater Or Equal?(x=w785, y=u16 1) -> (x >= y?=w787:bool)
                                n554 = And(x=w787, y=w790) -> (x .and. y?=w786:bool)
                                n555 = And(x=w786, y=w791) -> (x .and. y?=w781:bool)
                                n556 = case shown="True" w792 {
                                tunnel: w798 -> [w799 w802]
                                tunnel: w794 -> [_ w801]
                                frame False {
                                n557 = call "PumpStop.vi"("Pump Address"="j", "Pump COMM Port"=w799) -> ()  [unwired: 9 in, 1 out]
                                }
                                frame True {
                                n558 = call "PumpDispense.vi"("Flowrate(ul/min)"=w801, "Pump Address"="j", "Pump COMM Port"=w802) -> ()  [unwired: 7 in, 2 out]
                                }
                                }
                                n559 = Not Equal?(x=23.0, y=w779) -> (x != y?=w782:bool)
                                n560 = And(x=w782, y=w781) -> (x .and. y?=w780:bool)
                                n561 = case shown="True" w780 {
                                tunnel: w779 -> [_ w805]
                                frame False {
                                n562 = local write "Temperature Control 4"(FALSE ("Temperature Control 4")) -> ()
                                }
                                frame True {
                                n563 = local write "Temperature SP 4"(w805) -> ()
                                n564 = local write "Temperature Control 4"(TRUE ("Temperature Control 5")) -> ()
                                }
                                }
                                n565 = Wait (ms)(milliseconds to wait=u32 300) -> ()  [unwired: 1 out]
                              }
                              frame #4 {
                                # "Bay 5"
                                n566 = Index Array(array=w823, index=5) -> (element=w822:dbl)
                                n567 = Index Array(array=w823, index=4) -> (element=w810:dbl)
                                n568 = script code="MATLAB script"("T5_SP"=w810) -> ()  [unwired: 1 in, 1 out]
                                n569 = local read "BAY 5"() -> (w814:u16)
                                n570 = Not Equal To 0?(x=w822) -> (x != 0?=w821:bool)
                                n571 = And(x=w821, y=w819) -> (x .and. y?=w820:bool)
                                n572 = Less Or Equal?(x=w814, y=u16 4) -> (x <= y?=w818:bool)
                                n573 = Greater Or Equal?(x=w814, y=u16 1) -> (x >= y?=w815:bool)
                                n574 = case shown="False" w820 {
                                tunnel: w826 -> [w827 w830]
                                tunnel: w822 -> [_ w829]
                                frame False {
                                n575 = call "PumpStop.vi"("Pump Address"="h", "Pump COMM Port"=w827) -> ()  [unwired: 9 in, 1 out]
                                }
                                frame True {
                                n576 = call "PumpDispense.vi"("Flowrate(ul/min)"=w829, "Pump Address"="h", "Pump COMM Port"=w830) -> ()  [unwired: 7 in, 2 out]
                                }
                                }
                                n577 = And(x=w815, y=w818) -> (x .and. y?=w813:bool)
                                n578 = And(x=w813, y=w819) -> (x .and. y?=w808:bool)
                                n579 = Not Equal?(x=23.0, y=w810) -> (x != y?=w809:bool)
                                n580 = And(x=w809, y=w808) -> (x .and. y?=w807:bool)
                                n581 = case shown="True" w807 {
                                tunnel: w810 -> [_ w833]
                                frame False {
                                n582 = local write "Temperature Control 5"(FALSE ("Temperature Control 5")) -> ()
                                }
                                frame True {
                                n583 = local write "Temperature SP 5"(w833) -> ()
                                n584 = local write "Temperature Control 5"(TRUE ("Temperature Control 5")) -> ()
                                }
                                }
                                n585 = Wait (ms)(milliseconds to wait=u32 300) -> ()  [unwired: 1 out]
                              }
                            }
                          }
                          frame #1 {
                            # "Wait till Steady State temperature readings on all bays"
                            n586 = while {
                              tunnel: w836 -> [w837]
                              stop <- w838 stop-if-true
                              n587 = flat-sequence {
                                tunnel: [w841] -> w838
                                tunnel: w837 -> [w840]
                                frame #0 {
                                n588 = Wait (ms)(milliseconds to wait=u32 1500) -> ()  [unwired: 1 out]
                                }
                                frame #1 {
                                n589 = local read "Temp SS? 2"() -> (w844:bool)
                                n590 = local read "Temp SS? 3"() -> (w845:bool)
                                n591 = local read "Temp SS? 4"() -> (w846:bool)
                                n592 = local read "Temp SS? 5"() -> (w847:bool)
                                n593 = local read "Temp SS? 1"() -> (w843:bool)
                                n594 = Not(x=w840) -> (.not. x?=w853:bool)
                                n595 = local read "Stop"() -> (w842:bool)
                                n596 = And(x=w845, y=w846) -> (x .and. y?=w849:bool)
                                n597 = And(x=w843, y=w844) -> (x .and. y?=w850:bool)
                                n598 = And(x=w850, y=w849) -> (x .and. y?=w848:bool)
                                n599 = And(x=w848, y=w847) -> (x .and. y?=w851:bool)
                                n600 = Or(x=w853, y=w851) -> (x .or. y?=w852:bool)
                                n601 = Or(x=w852, y=w842) -> (x .or. y?=w841:bool)
                                }
                              }
                            }
                            n602 = local write "Calculate condition"(TRUE ("Calculate condition")) -> ()
                          }
                          frame #2 {
                            n603 = flat-sequence {
                              tunnel: w856 -> [w858]
                              tunnel: [w858] -> w855
                              tunnel: w855 -> [w865]
                              tunnel: [w865] -> w854
                              frame #0 {
                                n604 = local write "Equlibrating Temperature"(TRUE) -> ()
                              }
                              frame #1 {
                                # "Wait 1.5 system volumes"
                                n605 = local read "Number of System Flushes per condtion"() -> (w862:dbl)
                                n606 = local read "Extra system dead volume"() -> (w863:dbl)
                                n607 = script code="start = tic;\nP_tot = P1+P2+P3+P4+P5+P6;\nif P_tot >0\n  extra_res = extr_sys_dead_vol/P_tot;\nelse\n   extra_res =0;\nend\ntotal_sys_res = tau1 + tau2 + tau3 + tau4 + tau5 + extra_res;\ntotal_wait_time = total_sys_res*num_flush_per_cond*60;"("extr_sys_dead_vol"=w863, "num_flush_per_cond"=w862) -> ("??"=w866:errorcluster, "total_wait_time"=w860:dbl, "total_sys_res"=→"Total System Resisdence Time(min)":dbl)  [unwired: 1 in]
                                n608 = Divide(x=w860, y=60.0) -> (x/y=→"total_flush_time":dbl)
                                n609 = while {
                                tunnel: w865 -> [w868]
                                tunnel: w866 -> [w871]
                                stop <- w872 stop-if-true
                                # "Check if system is flushed every 10 seconds"
                                n610 = script code="end1 = toc(start);\nflush_time = 0;\nif end1 > total_wait_time\n   flush_time = 1;\nend\ncurr_wait_time = end1 /60;"("??"=w871) -> ("flush_time"=w875:dbl, "curr_wait_time"=w870:dbl)  [unwired: 1 out]
                                "curr_wait_time" <- w870
                                n611 = Not Equal To 0?(x=w875) -> (x != 0?=w874:bool)
                                n612 = Multiply(x=60.0, y=w870) -> ()  [unwired: 1 out]
                                n613 = local read "Stop"() -> (w877:bool)
                                n614 = Or(x=w874, y=w877) -> (x .or. y?=w873:bool)
                                n615 = Not(x=w868) -> (.not. x?=w867:bool)
                                n616 = Wait (ms)(milliseconds to wait=u32 10000) -> ()  [unwired: 1 out]
                                n617 = Or(x=w873, y=w867) -> (x .or. y?=w872:bool)
                                }
                              }
                            }
                          }
                          frame #3 {
                            # "Collect HPLC Data"
                            n618 = flat-sequence {
                              tunnel: w880 -> [w889]
                              tunnel: w879 -> [w888]
                              tunnel: w878 -> [w887]
                              tunnel: w878 -> [w886]
                              frame #0 {
                                n619 = local read "pause for ms"() -> (w883:bool)
                                n620 = case shown="True" w883 {
                                frame False {
                                }
                                frame True {
                                n621 = One Button Dialog(message="Press OK to Analyze Data", button name ("OK")="OK" ("Left Button Text (\"Yes\")")) -> ()  [unwired: 1 out]
                                }
                                }
                                n622 = local write "Flushing System"(TRUE ("Flushing System")) -> ()
                                "System Flushed?" <- TRUE ("System Flushed?")
                              }
                              frame #1 {
                                n623 = flat-sequence {
                                tunnel: w889 -> [w894]
                                tunnel: w888 -> [_]
                                tunnel: w887 -> [w893]
                                tunnel: w886 -> [w892]
                                frame #0 {
                                }
                                frame #1 {
                                n624 = flat-sequence {
                                tunnel: w894 -> [w896]
                                tunnel: w893 -> [w971]
                                tunnel: w894 -> [_]
                                tunnel: [w982] -> w891
                                tunnel: [w981] -> w890
                                tunnel: w892 -> [w980]
                                tunnel: w891 -> [w1002]
                                tunnel: w890 -> [w1001]
                                frame #0 {
                                n625 = local read "COMM Port :: Milligat Pumps"() -> (w898:refnum<visa-resource-name>)
                                n626 = stacked-sequence {
                                tunnel: w898 -> [w906 w918 w934 w939 w948 w961]
                                tunnel: w896 -> [w905 w914 w931 w941 w950 w957]
                                tunnel: 1.0 ("Flowrate(ul/min)") -> [w904 w913 w929 w938 w947 w956]
                                frame #0 {
                                n627 = Index Array(array=w905, index=0) -> (element=w908:dbl)
                                n628 = Greater Than 0?(x=w908) -> (x > 0?=w907:bool)
                                n629 = case shown="True" w907 {
                                tunnel: w906 -> [_ w911]
                                tunnel: w904 -> [_ w910]
                                frame False {
                                }
                                frame True {
                                n630 = call "PumpDispense.vi"("Flowrate(ul/min)"=w910, "Pump Address"="f", "Pump COMM Port"=w911) -> ()  [unwired: 7 in, 2 out]
                                }
                                }
                                }
                                frame #1 {
                                n631 = Index Array(array=w914, index=1) -> (element=w916:dbl)
                                n632 = Greater Than 0?(x=w916) -> (x > 0?=w915:bool)
                                n633 = case shown="True" w915 {
                                tunnel: w913 -> [_ w920]
                                tunnel: w918 -> [_ w919]
                                frame False {
                                }
                                frame True {
                                n634 = local read "Syringe_pump?"() -> (w921:bool)
                                n635 = case shown="True" w921 {
                                tunnel: w920 -> [w922 w927]
                                tunnel: w919 -> [w923 _]
                                frame False {
                                n636 = call "PumpDispense.vi"("Flowrate(ul/min)"=w922, "Pump Address"="g", "Pump COMM Port"=w923) -> ()  [unwired: 7 in, 2 out]
                                }
                                frame True {
                                w925 = u16 0 items=["uL/min", "uL/hr", "mL/min", "mL/hr"] ("Units")
                                n637 = local read "COMM Port:: Harvard Syringe Pump"() -> (w928:refnum<visa-resource-name>)
                                n638 = call <instrlib>:"WriteSP.vi"("VISA IN"=w928, "Pump Address"=i8 0, "SP"=w927, "Units"=w925) -> ()  [unwired: 5 in, 7 out]
                                }
                                }
                                }
                                }
                                }
                                frame #2 {
                                n639 = Index Array(array=w931, index=2) -> (element=w932:dbl)
                                n640 = Greater Than 0?(x=w932) -> (x > 0?=w930:bool)
                                n641 = case shown="True" w930 {
                                tunnel: w934 -> [_ w936]
                                tunnel: w929 -> [_ w935]
                                frame False {
                                }
                                frame True {
                                n642 = call "PumpDispense.vi"("Flowrate(ul/min)"=w935, "Pump Address"="i", "Pump COMM Port"=w936) -> ()  [unwired: 7 in, 2 out]
                                }
                                }
                                }
                                frame #3 {
                                n643 = Index Array(array=w941, index=3) -> (element=w942:dbl)
                                n644 = Greater Than 0?(x=w942) -> (x > 0?=w940:bool)
                                n645 = case shown="True" w940 {
                                tunnel: w939 -> [_ w945]
                                tunnel: w938 -> [_ w944]
                                frame False {
                                }
                                frame True {
                                n646 = call "PumpDispense.vi"("Flowrate(ul/min)"=w944, "Pump Address"="e", "Pump COMM Port"=w945) -> ()  [unwired: 7 in, 2 out]
                                }
                                }
                                }
                                frame #4 {
                                n647 = Index Array(array=w950, index=4) -> (element=w951:dbl)
                                n648 = Greater Than 0?(x=w951) -> (x > 0?=w949:bool)
                                n649 = case shown="True" w949 {
                                tunnel: w948 -> [_ w954]
                                tunnel: w947 -> [_ w953]
                                frame False {
                                }
                                frame True {
                                n650 = call "PumpDispense.vi"("Flowrate(ul/min)"=w953, "Pump Address"="j", "Pump COMM Port"=w954) -> ()  [unwired: 7 in, 2 out]
                                }
                                }
                                }
                                frame #5 {
                                n651 = Index Array(array=w957, index=5) -> (element=w959:dbl)
                                n652 = Greater Than 0?(x=w959) -> (x > 0?=w958:bool)
                                n653 = case shown="True" w958 {
                                tunnel: w961 -> [_ w963]
                                tunnel: w956 -> [_ w962]
                                frame False {
                                }
                                frame True {
                                n654 = call "PumpDispense.vi"("Flowrate(ul/min)"=w962, "Pump Address"="h", "Pump COMM Port"=w963) -> ()  [unwired: 7 in, 2 out]
                                }
                                }
                                }
                                }
                                n655 = stacked-sequence {
                                tunnel: FALSE -> [w899 w900 w901 w902 w903]
                                frame #0 {
                                n656 = local write "Temperature Control 1"(w899) -> ()
                                }
                                frame #1 {
                                n657 = local write "Temperature Control 2"(w900) -> ()
                                }
                                frame #2 {
                                n658 = local write "Temperature Control 3"(w901) -> ()
                                }
                                frame #3 {
                                n659 = local write "Temperature Control 4"(w902) -> ()
                                }
                                frame #4 {
                                n660 = local write "Temperature Control 5"(w903) -> ()
                                }
                                }
                                }
                                frame #1 {
                                n661 = while {
                                stop <- w970 stop-if-true
                                n662 = local read "Phase_Sensor_voltage"() -> (w965:dbl)
                                n663 = script code="organic_phase = 0;\nif start_phase_time \n   start_phase_timer = tic;\n   start_phase_time = 0;\nelse\n  %ignore phase sensor values\n  %if not(phase_sensor_val >2.9 && phase_sensor_val <3.8)\n    %    start_phase_timer = tic;\n   %end\n\n   end_phase_time =  toc(start_phase_timer )\n\n   if end_phase_time > 2\n       organic_phase = 1;\n       start_phase_time = 1;\n   end\n\nend"("phase_sensor_val"=w965) -> ("organic_phase"=w967:dbl)  [unwired: 1 in, 1 out]
                                n664 = local read "Stop"() -> (w969:bool)
                                n665 = Not Equal To 0?(x=w967) -> (x != 0?=w968:bool)
                                n666 = Or(x=w968, y=w969) -> (x .or. y?=w970:bool)
                                n667 = Wait (ms)(milliseconds to wait=u32 300) -> ()  [unwired: 1 out]
                                }
                                }
                                frame #2 {
                                n668 = local read "Stop"() -> (w973:bool)
                                n669 = Not(x=w973) -> (.not. x?=w972:bool)
                                n670 = local read "Sample Valve COMM::Port"() -> (w974:refnum<visa-resource-name>)
                                n671 = case shown="True" w972 {
                                tunnel: w974 -> [_ w976]
                                tunnel: w971 -> [_ w975]
                                frame False {
                                }
                                frame True {
                                n672 = flat-sequence {
                                tunnel: w975 -> [_]
                                tunnel: w976 -> [w979]
                                frame #0 {
                                n673 = local read "Sample Valve COMM::Port"() -> (w977:refnum<visa-resource-name>)
                                n674 = call "NanoValve Inject.vi"("VISA resource name"=w977) -> ()  [unwired: 10 in, 1 out]
                                }
                                frame #1 {
                                n675 = Wait (ms)(milliseconds to wait=u32 1000) -> ()  [unwired: 1 out]
                                }
                                frame #2 {
                                n676 = call "NanoValve Load.vi"("VISA resource name"=w979) -> ()  [unwired: 10 in, 1 out]
                                }
                                }
                                }
                                }
                                }
                                frame #3 {
                                n677 = local read "Stop"() -> (w985:bool)
                                n678 = local read "Bay Parameters"() -> (w981:T2)
                                n679 = Unbundle By Name(w981) -> ("Hplc Wait time(min)"=w983:dbl)
                                n680 = Not(x=w985) -> (.not. x?=w984:bool)
                                n681 = case shown="True" w984 {
                                tunnel: w983 -> [_ w989]
                                tunnel: [errorcluster {"status"=FALSE, "code"=0, "source"=""} ("error out") w987] -> w982
                                tunnel: w981 -> [_ _]
                                tunnel: w980 -> [_ w988]
                                frame False {
                                }
                                frame True {
                                n682 = flat-sequence {
                                tunnel: w989 -> [_]
                                tunnel: w988 -> [_]
                                tunnel: [w991] -> w987
                                frame #0 {
                                # "Wait till for MS Method"
                                n683 = script code="Conc =0;"() -> ()  [unwired: 1 in, 1 out]
                                }
                                frame #1 {
                                n684 = Tick Count (ms)() -> (millisecond timer value=w990:u32)
                                n685 = while {
                                tunnel: [w997] -> w991
                                tunnel: w990 -> [w992]
                                stop <- w1000 stop-if-true
                                n686 = script code="Conc = Conc - MS_Data(1);"() -> ("??"=w997:errorcluster)  [unwired: 1 in]
                                n687 = Tick Count (ms)() -> (millisecond timer value=w996:u32)
                                n688 = Subtract(x=w996, y=w992) -> (x-y=w995:u32)
                                n689 = local read "Stop"() -> (w999:bool)
                                n690 = Greater?(x=w995, y=u32 80000) -> (0:w993:bool)
                                n691 = Or(x=w993, y=w999) -> (x .or. y?=w1000:bool)
                                n692 = Wait (ms)(milliseconds to wait=u32 300) -> ()  [unwired: 1 out]
                                }
                                }
                                }
                                }
                                }
                                }
                                frame #4 {
                                n693 = Unbundle By Name(w1002) -> ("status"=w1003:bool)
                                n694 = case shown="False" w1003 {
                                tunnel: w1001 -> [_ w1004]
                                frame False {
                                }
                                frame True {
                                n695 = while {
                                tunnel: w1004 -> [w1006]
                                stop <- w1005 stop-if-true
                                w1011 = "An error occured while trying to read HPLC data. " ("message")
                                n696 = local write "Error Message"(w1011) -> ()
                                n697 = call <vilib>:"Three Button Dialog.vi"("Right Button Text (\"Cancel\")"="STOP EXPs" ("F button name (\"Cancel\")"), "Center Button Text (\"No\")"="REDO" ("T button name (\"OK\")"), "Left Button Text (\"Yes\")"="REREAD" ("T button name (\"OK\")"), "message"=w1011) -> ("Which Button?"=w1007:T19)  [unwired: 7 in]
                                n698 = case shown="\"Left Button\"" w1007 {
                                tunnel: w1006 -> [_ _ w1018 _]
                                tunnel: [TRUE TRUE w1017 w1020] -> w1005
                                frame "Right Button" {
                                w1012 = TRUE ("Setup Error")
                                n699 = local write "System Error"(w1012) -> ()
                                n700 = local write "Setup Error"(w1012) -> ()
                                n701 = script code="system_error = 1"() -> ()  [unwired: 1 in, 1 out]
                                n702 = local write "Stop"(w1012) -> ()
                                }
                                frame "Center Button" {
                                n703 = script code="redo = true;\nopt_ctr = 1;\nCurrExp = CurrExp + 1;\nncall0 = ncall0 +1;\nif req_ctr == req_tot\n       opt_ctr = 3;\n  else\n     req_ctr = req_ctr +1;\nend"() -> ()  [unwired: 1 in, 1 out]
                                }
                                frame "Left Button" {
                                n704 = Unbundle By Name(w1018) -> ("hplc File Name"=w1019:string)
                                n705 = call "hplc_analyze.vi"("File Path"=w1019) -> ("error out"=w1015:errorcluster)  [unwired: 10 in]
                                n706 = Unbundle By Name(w1015) -> ("status"=w1016:bool)
                                n707 = Not(x=w1016) -> (.not. x?=w1017:bool)
                                }
                                frame "Window Close" {
                                w1020 = TRUE
                                n708 = local write "Setup Error"(w1020) -> ()
                                n709 = script code="system_error = 1"() -> ()  [unwired: 1 in, 1 out]
                                n710 = local write "Stop"(w1020) -> ()
                                }
                                }
                                }
                                }
                                }
                                }
                                frame #5 {
                                n711 = disable-structure shown="Disabled" {
                                frame Disabled {
                                n712 = flat-sequence {
                                tunnel: w1022 -> [w1027]
                                tunnel: [w1027] -> w1021
                                frame #0 {
                                n713 = Wait (ms)(milliseconds to wait=u32 500) -> ()  [unwired: 1 out]
                                }
                                }
                                n714 = call-poly <vilib>:"Digital Write.vi"("Output Value"=FALSE, "DO Channel"=u8 22) -> ("LINX Resource"=w1022:T10)  [unwired: 8 in, 1 out]
                                n715 = call-poly <vilib>:"Digital Write.vi"("Output Value"=TRUE, "DO Channel"=u8 22, "LINX Resource"=w1021) -> ()  [unwired: 7 in, 2 out]
                                }
                                frame Enabled {
                                }
                                }
                                }
                                }
                                }
                                }
                              }
                              frame #2 {
                                n716 = local read "Stop"() -> (w1030:bool)
                                n717 = local write "HPLC Analysis"(TRUE ("HPLC Analysis")) -> ()
                                n718 = Not(x=w1030) -> (.not. x?=w1029:bool)
                                n719 = case shown="True" w1029 {
                                frame False {
                                }
                                frame True {
                                n720 = script code="C_measured =Conc;\nFvalues(end +1,:) = [Conc];"() -> ()  [unwired: 1 in, 1 out]
                                }
                                }
                              }
                            }
                          }
                          frame #4 {
                            n721 = local read "Stop"() -> (w1033:bool)
                            n722 = Not(x=w1033) -> (.not. x?=w1032:bool)
                            n723 = case shown="True" w1032 {
                              tunnel: [1.0 w1044] -> w1034
                              frame False {
                              }
                              frame True {
                                # "Save data to excel file"
                                n724 = local read "Bay Parameters"() -> (w1042:T2)
                                n725 = Unbundle By Name(w1042) -> ("Total Number of Experiments 2"=w1041:dbl)
                                n726 = script code="analyze_labview_results"("ncall"=w1041) -> ("terminate"=w1044:dbl, "ncall0"=w1043:dbl, "experiment_history"=w1039:dbl[][], "Pbest"=w1037:dbl[], "Tbest"=w1038:dbl[], "best_exp_num"=w1036:dbl)  [unwired: 1 in, 1 out]
                                n727 = local write "Flowrates(ul/min)_best"(w1037) -> ()
                                n728 = local write "temperature_best"(w1038) -> ()
                                n729 = local write "best_exp_num"(w1036) -> ()
                                n730 = local write "Current Experiment"(w1043) -> ()
                                n731 = local write "Total Number of Experiments"(w1041) -> ()
                                n732 = call-poly <vilib>:"Array To Matrix.vi"("Real 2D Array"=w1039) -> ("Real Matrix"=w1040:T18)
                                n733 = local write "experiment history"(w1040) -> ()
                              }
                            }
                          }
                          frame #5 {
                            n734 = local read "Num_exp_till_pause"() -> (w1046:i32)
                            n735 = Increment(x=w1046) -> (x+1=w1045:i32)
                            n736 = local write "Num_exp_till_pause"(w1045) -> ()
                          }
                          frame #6 {
                            # "Pause System"
                            n737 = local read "Bay Parameters"() -> (w1054:T2)
                            n738 = Unbundle By Name(w1054) -> ("Num_conditons_per_wait"=w1053:dbl)
                            n739 = local read "Num_exp_till_pause"() -> (w1052:i32)
                            n740 = Equal?(x=w1053, y=w1052) -> (x = y?=w1051:bool)
                            n741 = local read "Run_Stop_cluster"() -> (w1048:T7)
                            n742 = Unbundle By Name(w1048) -> ("Stop Run Button"=w1050:bool)
                            n743 = Or(x=w1050, y=w1051) -> (x .or. y?=w1049:bool)
                            n744 = case shown="True" w1049 {
                              tunnel: w1053 -> [w1057 _]
                              tunnel: w1052 -> [w1058 _]
                              tunnel: w1048 -> [_ w1060]
                              frame False {
                                n745 = Greater?(x=w1058, y=w1057) -> (0:w1056:bool)
                                n746 = case shown="True" w1056 {
                                frame False {
                                }
                                frame True {
                                n747 = local write "Num_exp_till_pause"(0 ("Num_exp_till_pause")) -> ()
                                }
                                }
                              }
                              frame True {
                                n748 = flat-sequence {
                                tunnel: w1060 -> [w1089]
                                frame #0 {
                                w1064 = string[] ["e", "f", "g", "h", "i", "j"]
                                # "Turn off pumps and stop controling temperature"
                                n749 = stacked-sequence {
                                frame #0 {
                                n750 = local write "Temperature Control 1"(FALSE ("Temperature Control 1")) -> ()
                                }
                                frame #1 {
                                n751 = local write "Temperature Control 2"(FALSE ("Temperature Control 2")) -> ()
                                }
                                frame #2 {
                                n752 = local write "Temperature Control 3"(FALSE ("Temperature Control 3")) -> ()
                                }
                                frame #3 {
                                n753 = local write "Temperature Control 4"(FALSE ("Temperature Control 4")) -> ()
                                }
                                frame #4 {
                                n754 = local write "Temperature Control 5"(FALSE ("Temperature Control 5")) -> ()
                                }
                                }
                                n755 = local read "COMM Port:: Harvard Syringe Pump"() -> (w1062:refnum<visa-resource-name>)
                                n756 = local read "Syringe_pump?"() -> (w1061:bool)
                                n757 = local read "COMM Port :: Milligat Pumps"() -> (w1063:refnum<visa-resource-name>)
                                n758 = Array Size(array=w1064) -> (size(s)=w1065:i32)
                                n759 = case shown="True" w1061 {
                                tunnel: w1062 -> [_ w1074]
                                frame False {
                                }
                                frame True {
                                n760 = call <instrlib>:"Stop.vi"("VISA IN"=w1074, "Pump Address"=i8 0) -> ()  [unwired: 7 in, 7 out]
                                }
                                }
                                n761 = for {
                                N: w1065 -> [_]
                                tunnel: w1064 -> [w1071] mode=indexing
                                tunnel: w1063 -> [w1072]
                                n762 = call "PumpStop.vi"("Pump Address"=w1071, "Pump COMM Port"=w1072) -> ()  [unwired: 9 in, 1 out]
                                }
                                }
                                frame #1 {
                                n763 = local read "Stop"() -> (w1077:bool)
                                n764 = Not(x=w1077) -> (.not. x?=w1076:bool)
                                n765 = case shown="True" w1076 {
                                frame False {
                                }
                                frame True {
                                n766 = while {
                                stop <- w1083 stop-if-true
                                # "Wait till user confirms system resume"
                                n767 = Two Button Dialog(message="System is currently paused. Refill Syringes, flush lines, then press OK to continue optimization.\nOr Redo to repeat condition ", 1:"REDO" ("F button name (\"Cancel\")"), 2:"OK" ("Left Button Text (\"Yes\")")) -> (T button?=w1079:bool)
                                n768 = case shown="False" w1079 {
                                tunnel: [TRUE TRUE] -> w1078
                                frame False {
                                n769 = script code="redo = true;"() -> ()  [unwired: 1 in, 1 out]
                                }
                                frame True {
                                }
                                }
                                n770 = local read "Stop"() -> (w1084:bool)
                                n771 = Or(x=w1078, y=w1084) -> (x .or. y?=w1083:bool)
                                }
                                }
                                }
                                n772 = local write "stop_xl_write"(TRUE ("stop_xl_write")) -> ()
                                }
                                frame #2 {
                                n773 = local write "Num_exp_till_pause"(0 ("Num_exp_till_pause")) -> ()
                                n774 = Bundle By Name(cluster=w1089, "Stop Run Button"=FALSE) -> (w1087:T7)
                                n775 = local write "Run_Stop_cluster"(w1087) -> ()
                                }
                                }
                              }
                            }
                          }
                          frame #7 {
                            w1092 = FALSE
                            n776 = local write "Equlibrating Temperature"(w1092) -> ()
                            n777 = local write "Calculate condition"(w1092) -> ()
                            n778 = local write "Flushing System"(w1092) -> ()
                            n779 = local write "HPLC Analysis"(w1092) -> ()
                            n780 = local write "stop_xl_write"(TRUE ("stop_xl_write")) -> ()
                          }
                        }
                        n781 = while {
                          stop <- w1119 stop-if-true
                          n782 = flat-sequence {
                            frame #0 {
                              n783 = script code="save_excel_time_data;"() -> ()  [unwired: 1 in, 1 out]
                            }
                            frame #1 {
                              n784 = Wait (ms)(milliseconds to wait=u32 30000) -> ()  [unwired: 1 out]
                            }
                          }
                          n785 = local read "Stop"() -> (w1120:bool)
                          n786 = local read "stop_xl_write"() -> (w1118:bool)
                          n787 = Or(x=w1118, y=w1120) -> (x .or. y?=w1119:bool)
                        }
                      }
                    }
                  }
                }
                n788 = Greater?(x=w608, y=w609) -> (0:w616:bool)
                n789 = Equal?(x=w614, y=1.0) -> (x = y?=w610:bool)
                n790 = local read "Stop"() -> (w617:bool)
                n791 = Or(x=w617, y=w616) -> (x .or. y?=w613:bool)
                n792 = Or(x=w610, y=w613) -> (x .or. y?=w612:bool)
                n793 = case shown="True" w610 {
                  frame False {
                  }
                  frame True {
                    w621 = u16 2 items=["System  Error", "System Running", "System Standby"] ("System Status")
                    n794 = local write "Stop"(TRUE ("Stop")) -> ()
                    n795 = local write "System Status"(w621) -> ()
                  }
                }
                "Optimization_loop_index" <- w618
              }
            }
          }
          n796 = while {
            tunnel: w596 -> [w1215]
            stop <- w1218 stop-if-true
            n797 = local read "Temperature Control 3"() -> (w1216:bool)
            n798 = local read "running?"() -> (w1214:bool)
            n799 = And(x=w1214, y=w1216) -> (x .and. y?=w1217:bool)
            n800 = case shown="True" w1217 {
              tunnel: w1215 -> [_ w1221]
              frame False {
                n801 = local write "Temp SS? 3"(TRUE) -> ()
              }
              frame True {
                # "Bay 3 Temperature Controller"
                n802 = local read "Temperature SP 3"() -> (w1222:dbl)
                n803 = local read "Temperature 3"() -> (w1225:dbl)
                n804 = Subtract(x=w1225, y=w1222) -> (x-y=w1234:dbl)
                n805 = Absolute Value(x=w1234) -> (abs(x)=w1236:dbl)
                n806 = Less Or Equal?(x=w1236, y=1.2) -> (x <= y?=w1233:bool)
                n807 = local write "Temp SS? 3"(w1233) -> ()
                n808 = local read "SSR Duration 3"() -> (w1243:dbl)
                n809 = call-poly <vilib>:"PID Online Autotuning.vi"("setpoint"=w1222, "manipulated variable"=w1243, "autotuning parameters"=T9 {"type of controller"=enum."PID", "relay cycles"=3, "relay amplitude"=1.0, "control specifications"=enum."Normal", "PV noise level"=0.1} ("Autotuning Parameters R1"), "process variable"=w1225, "PID gains in"=T8 {"Proportional gain Kc"=0.38538, "Integral time Ti (sec)"=0.524375, "Derivative time Ti (sec)"=0.12585} ("PID gains 2")) -> ("setpoint out"=w1241:dbl, "process variable out"=w1242:dbl, "PID gains out"=w1245:T17)  [unwired: 6 in, 2 out]
                n810 = Greater?(x=w1222, y=w1225) -> (0:w1232:bool)
                n811 = call <vilib>:"PID Autotuning (Temperature).vi"("desired temperature"=w1241, "measured temperature"=w1242, "PID gains in"=w1245, "output range"=cluster{"output high":dbl, "output low":dbl} {"output high"=3.0, "output low"=-1.0} ("Output range")) -> ("output"=w1238:dbl)  [unwired: 12 in, 3 out]
                n812 = Multiply(x=1000.0, y=w1238) -> (x*y=w1240:dbl)
                n813 = local write "SSR Duration 3"(w1238) -> ()
                n814 = Greater Than 0?(x=w1240) -> (x > 0?=w1231:bool)
                n815 = And(x=w1231, y=w1232) -> (x .and. y?=w1229:bool)
                n816 = Subtract(x=w1225, y=10.0) -> (x-y=w1227:dbl)
                n817 = Less?(x=w1227, y=w1222) -> (x < y?=w1230:bool)
                n818 = And(x=w1230, y=w1229) -> (x .and. y?=w1228:bool)
                n819 = case shown="True" w1228 {
                  tunnel: [errorcluster {"status"=FALSE, "code"=0, "source"=""} ("error out") w1257] -> _
                  tunnel: 4 -> [_ w1255]
                  tunnel: w1240 -> [w1251 w1256]
                  tunnel: [0.0 w1259] -> w1223
                  tunnel: w1222 -> [_ w1258]
                  tunnel: w1221 -> [_ w1254]
                  frame False {
                    n820 = Absolute Value(x=w1251) -> (abs(x)=w1252:dbl)
                    n821 = Wait (ms)(milliseconds to wait=w1252) -> ()  [unwired: 1 out]
                  }
                  frame True {
                    n822 = call "TurnOnRelayArduino.vi"("channel"=w1255, "duration"=w1256, "LINX Resource"=w1254) -> ("error out"=w1257:errorcluster)  [unwired: 7 in, 1 out]
                    n823 = script code="tempdiff3= SP3 - T3;\nif tempdiff3 > 10\n  if slope3 < .01\n     temp_check3 = temp_check3 + 1;\n  else\n      temp_check3 =0;\n  end\nend\n\nif temp_check3 > 9\n  temp_error3 = 1\nend"("SP3"=w1258) -> ("temp_error3"=w1259:dbl)  [unwired: 1 in, 1 out]
                  }
                }
                n824 = Not Equal To 0?(x=w1223) -> (x != 0?=w1224:bool)
                n825 = case shown="True" w1224 {
                  frame False {
                  }
                  frame True {
                    n826 = local write "Error Message"("Bay 3 Temperature Heating Error") -> ()
                  }
                }
                n827 = case shown="True" w1224 {
                  tunnel: w1224 -> [_ w1249]
                  frame False {
                  }
                  frame True {
                    n828 = local write "System Error"(w1249) -> ()
                    n829 = local write "Stop"(w1249) -> ()
                  }
                }
              }
            }
            n830 = Wait (ms)(milliseconds to wait=u32 400) -> ()  [unwired: 1 out]
            n831 = local read "Stop"() -> (w1218:bool)
          }
          n832 = while {
            tunnel: w596 -> [w1169]
            stop <- w1172 stop-if-true
            n833 = local read "running?"() -> (w1168:bool)
            n834 = Wait (ms)(milliseconds to wait=u32 400) -> ()  [unwired: 1 out]
            n835 = local read "Temperature Control 4"() -> (w1171:bool)
            n836 = And(x=w1168, y=w1171) -> (x .and. y?=w1170:bool)
            n837 = case shown="True" w1170 {
              tunnel: w1169 -> [_ w1175]
              frame False {
                n838 = local write "Temp SS? 4"(TRUE ("Temp SS? 4")) -> ()
              }
              frame True {
                # "Bay 4 Temperature Controller"
                n839 = local read "Temperature SP 4"() -> (w1178:dbl)
                n840 = local read "Temperature 4"() -> (w1181:dbl)
                n841 = Subtract(x=w1181, y=w1178) -> (x-y=w1188:dbl)
                n842 = Absolute Value(x=w1188) -> (abs(x)=w1190:dbl)
                n843 = Less Or Equal?(x=w1190, y=1.2) -> (x <= y?=w1187:bool)
                n844 = local write "Temp SS? 4"(w1187) -> ()
                n845 = local read "SSR Duration 4"() -> (w1191:dbl)
                n846 = call-poly <vilib>:"PID Online Autotuning.vi"("setpoint"=w1178, "manipulated variable"=w1191, "autotuning parameters"=T9 {"type of controller"=enum."PID", "relay cycles"=3, "relay amplitude"=1.0, "control specifications"=enum."Normal", "PV noise level"=0.1} ("Autotuning Parameters R1"), "process variable"=w1181, "PID gains in"=T8 {"Proportional gain Kc"=0.38538, "Integral time Ti (sec)"=0.524375, "Derivative time Ti (sec)"=0.12585} ("PID gains 2")) -> ("setpoint out"=w1193:dbl, "process variable out"=w1194:dbl, "PID gains out"=w1196:T17)  [unwired: 6 in, 2 out]
                n847 = call <vilib>:"PID Autotuning (Temperature).vi"("desired temperature"=w1193, "measured temperature"=w1194, "PID gains in"=w1196, "output range"=cluster{"output high":dbl, "output low":dbl} {"output high"=3.0, "output low"=-1.0} ("Output range")) -> ("output"=w1192:dbl)  [unwired: 12 in, 3 out]
                n848 = Subtract(x=w1181, y=10.0) -> (x-y=w1180:dbl)
                n849 = Less?(x=w1180, y=w1178) -> (x < y?=w1182:bool)
                n850 = Multiply(x=1000.0, y=w1192) -> (x*y=w1200:dbl)
                n851 = Greater?(x=w1178, y=w1181) -> (0:w1186:bool)
                n852 = Greater Than 0?(x=w1200) -> (x > 0?=w1185:bool)
                n853 = local write "SSR Duration 4"(w1192) -> ()
                n854 = And(x=w1185, y=w1186) -> (x .and. y?=w1184:bool)
                n855 = And(x=w1182, y=w1184) -> (x .and. y?=w1183:bool)
                n856 = case shown="True" w1183 {
                  tunnel: [errorcluster {"status"=FALSE, "code"=0, "source"=""} ("error out") w1211] -> _
                  tunnel: 5 -> [_ w1209]
                  tunnel: w1200 -> [w1205 w1210]
                  tunnel: w1178 -> [_ w1213]
                  tunnel: [0.0 w1212] -> w1177
                  tunnel: w1175 -> [_ w1208]
                  frame False {
                    n857 = Absolute Value(x=w1205) -> (abs(x)=w1206:dbl)
                    n858 = Wait (ms)(milliseconds to wait=w1206) -> ()  [unwired: 1 out]
                  }
                  frame True {
                    n859 = call "TurnOnRelayArduino.vi"("channel"=w1209, "duration"=w1210, "LINX Resource"=w1208) -> ("error out"=w1211:errorcluster)  [unwired: 7 in, 1 out]
                    n860 = script code="tempdiff4= SP4 - T4;\nif tempdiff4 > 10\n  if slope4 < .01\n     temp_check4 = temp_check4 + 1;\n  else\n      temp_check4 =0;\n  end\nend\n\nif temp_check4 > 9\n  temp_error4 = 1\nend"("SP4"=w1213) -> ("temp_error4"=w1212:dbl)  [unwired: 1 in, 1 out]
                  }
                }
                n861 = Not Equal To 0?(x=w1177) -> (x != 0?=w1176:bool)
                n862 = case shown="True" w1176 {
                  frame False {
                  }
                  frame True {
                    n863 = local write "Error Message"("Bay 4 Temperature Heating Error") -> ()
                  }
                }
                n864 = case shown="True" w1176 {
                  tunnel: w1176 -> [_ w1203]
                  frame False {
                  }
                  frame True {
                    n865 = local write "System Error"(w1203) -> ()
                    n866 = local write "Stop"(w1203) -> ()
                  }
                }
              }
            }
            n867 = local read "Stop"() -> (w1172:bool)
          }
          n868 = while {
            stop <- w601 stop-if-true
            n869 = script code="TempArr1=circshift(TempArr1,9);\nTempArr2=circshift(TempArr2,9);\nTempArr3=circshift(TempArr3,9);\nTempArr4=circshift(TempArr4,9);\nTempArr5=circshift(TempArr5,9);\n\nTempArr1(10)=T1;\nTempArr2(10)=T2;\nTempArr3(10)=T3;\nTempArr4(10)=T4;\nTempArr5(10)=T5;\n\n[slope1 temp] = polyfit([1,2,3,4,5,6,7,8,9,10]',TempArr1,1);\nslope1 = slope1(1);\n[slope2 temp] = polyfit([1,2,3,4,5,6,7,8,9,10]',TempArr2,1);\nslope2= slope2(1);\n[slope3 temp] = polyfit([1,2,3,4,5,6,7,8,9,10]',TempArr3,1);\nslope3 = slope3(1);\n[slope4 temp] = polyfit([1,2,3,4,5,6,7,8,9,10]',TempArr4,1);\nslope4 = slope4(1);\n[slope5 temp] = polyfit([1,2,3,4,5,6,7,8,9,10]',TempArr5,1);\nslope5 = slope5(1);"() -> ()  [unwired: 1 in, 1 out]
            n870 = Wait (ms)(milliseconds to wait=u32 600) -> ()  [unwired: 1 out]
            n871 = local read "Stop"() -> (w601:bool)
          }
          n872 = while {
            tunnel: w596 -> [w1123]
            stop <- w1126 stop-if-true
            n873 = local read "running?"() -> (w1122:bool)
            n874 = local read "Temperature Control 5"() -> (w1124:bool)
            n875 = And(x=w1122, y=w1124) -> (x .and. y?=w1125:bool)
            n876 = case shown="True" w1125 {
              tunnel: w1123 -> [_ w1129]
              frame False {
                n877 = local write "Temp SS? 5"(TRUE ("Temp SS? 5")) -> ()
              }
              frame True {
                # "Bay 5 Temperature Controller"
                n878 = local read "SSR Duration 5"() -> (w1145:dbl)
                n879 = local read "Temperature SP 5"() -> (w1131:dbl)
                n880 = local read "Temperature 5"() -> (w1134:dbl)
                n881 = Subtract(x=w1134, y=w1131) -> (x-y=w1142:dbl)
                n882 = Absolute Value(x=w1142) -> (abs(x)=w1144:dbl)
                n883 = Less Or Equal?(x=w1144, y=1.2) -> (x <= y?=w1141:bool)
                n884 = local write "Temp SS? 5"(w1141) -> ()
                n885 = call-poly <vilib>:"PID Online Autotuning.vi"("setpoint"=w1131, "manipulated variable"=w1145, "autotuning parameters"=T9 {"type of controller"=enum."PID", "relay cycles"=3, "relay amplitude"=1.0, "control specifications"=enum."Normal", "PV noise level"=0.1} ("Autotuning Parameters R1"), "process variable"=w1134, "PID gains in"=T8 {"Proportional gain Kc"=0.38538, "Integral time Ti (sec)"=0.524375, "Derivative time Ti (sec)"=0.12585} ("PID gains 2")) -> ("setpoint out"=w1147:dbl, "process variable out"=w1148:dbl, "PID gains out"=w1150:T17)  [unwired: 6 in, 2 out]
                n886 = call <vilib>:"PID Autotuning (Temperature).vi"("desired temperature"=w1147, "measured temperature"=w1148, "PID gains in"=w1150, "output range"=cluster{"output high":dbl, "output low":dbl} {"output high"=3.0, "output low"=-1.0} ("Output range")) -> ("output"=w1146:dbl)  [unwired: 12 in, 3 out]
                n887 = Multiply(x=1000.0, y=w1146) -> (x*y=w1154:dbl)
                n888 = Greater?(x=w1131, y=w1134) -> (0:w1139:bool)
                n889 = Greater Than 0?(x=w1154) -> (x > 0?=w1140:bool)
                n890 = local write "SSR Duration 5"(w1146) -> ()
                n891 = And(x=w1140, y=w1139) -> (x .and. y?=w1137:bool)
                n892 = Subtract(x=w1134, y=10.0) -> (x-y=w1135:dbl)
                n893 = Greater?(x=w1135, y=w1131) -> (0:w1138:bool)
                n894 = And(x=w1138, y=w1137) -> (x .and. y?=w1136:bool)
                n895 = case shown="True" w1136 {
                  tunnel: [errorcluster {"status"=FALSE, "code"=0, "source"=""} ("error out") w1165] -> _
                  tunnel: 6 -> [_ w1162]
                  tunnel: w1154 -> [w1159 w1163]
                  tunnel: [0.0 w1167] -> w1132
                  tunnel: w1131 -> [_ w1166]
                  tunnel: w1129 -> [_ w1164]
                  frame False {
                    n896 = Absolute Value(x=w1159) -> (abs(x)=w1160:dbl)
                    n897 = Wait (ms)(milliseconds to wait=w1160) -> ()  [unwired: 1 out]
                  }
                  frame True {
                    n898 = call "TurnOnRelayArduino.vi"("channel"=w1162, "duration"=w1163, "LINX Resource"=w1164) -> ("error out"=w1165:errorcluster)  [unwired: 7 in, 1 out]
                    n899 = script code="tempdiff5= SP5 - T5;\n\nif tempdiff5 > 10\n  if slope5 < .01\n     temp_check5 = temp_check5 + 1;\n  else\n      temp_check5 =0;\n  end\nend\n\nif temp_check5 >9\n  temp_error5 = 1\nend"("SP5"=w1166) -> ("temp_error5"=w1167:dbl)  [unwired: 1 in, 1 out]
                  }
                }
                n900 = Not Equal To 0?(x=w1132) -> (x != 0?=w1130:bool)
                n901 = case shown="True" w1130 {
                  frame False {
                  }
                  frame True {
                    n902 = local write "Error Message"("Bay 5 Temperature Heating Error") -> ()
                  }
                }
                n903 = case shown="True" w1130 {
                  tunnel: w1130 -> [_ w1157]
                  frame False {
                  }
                  frame True {
                    n904 = local write "Stop"(w1157) -> ()
                    n905 = local write "System Error"(w1157) -> ()
                  }
                }
              }
            }
            n906 = Wait (ms)(milliseconds to wait=u32 400) -> ()  [unwired: 1 out]
            n907 = local read "Stop"() -> (w1126:bool)
          }
        }
      }
      n908 = local read "IR Sensor Device"() -> (w63:T6)
      n909 = while {
        tunnel: errorcluster {"status"=FALSE, "code"=0, "source"=""} ("error out") -> [w139]
        tunnel: w63 -> [w158]
        stop <- w179 stop-if-true
        w136 = u8 7 items=["RAM IR raw  Ch1"=4, "RAM IR raw  Ch2"=5, "RAM T_A"=6, "RAM T_OBJ1"=7, "RAM T_OBJ2"=8, "EEPROM_To_max"=32, "EEPROM_To_min"=33, "EEPROM_PWM_CTRL"=34, "EEPROM_Ta_range"=35, "EEPROM_Emissivity_CorrCoeff"=36, "EEPROM_SMBus Address"=46, "EEPROM_ConfigReg"=37] ("Melexis_Cmmds")
        # "Bay 5 Temperature Read"
        # "Bay 4 Temperature Read"
        # "Bay 3 Temperature Read"
        # "Bay 2 Temperature Read"
        # "Bay 1 Temperature Read"
        n910 = local read "Stop"() -> (w179:bool)
        n911 = call "IRSensorNIRead.vi"("error in (no error)"=w139, "Melexis_Cmmds"=w136, "Address"=u8 1, "device reference"=w158) -> ("error out"=w161:errorcluster, "Temperature"=w159:dbl, "device reference out"=w157:T6)  [unwired: 5 in]
        n912 = local write "error out"(w161) -> ()
        n913 = Unbundle By Name(w161) -> ("status"=w160:bool)
        n914 = call-poly <vilib>:"PID Control Input Filter.vi"("input"=w159) -> ("output"=w172:dbl)  [unwired: 4 in]
        n915 = case shown="False" w160 {
          tunnel: w171 -> [w188 _]
          tunnel: [w188 w189] -> w176
          frame False {
            n916 = local write "Temperature 1"(w188) -> ()
          }
          frame True {
            n917 = local read "Temperature 1"() -> (w189:dbl)
          }
        }
        n918 = flat-sequence {
          tunnel: w172 -> [w202]
          tunnel: [w202] -> w171
          tunnel: w157 -> [w201]
          tunnel: [w201] -> w156
          frame #0 {
            n919 = Wait (ms)(milliseconds to wait=u32 100) -> ()  [unwired: 1 out]
          }
        }
        n920 = call "IRSensorNIRead.vi"("error in (no error)"=w139, "Melexis_Cmmds"=w136, "Address"=u8 2, "device reference"=w156) -> ("error out"=w148:errorcluster, "Temperature"=w149:dbl, "device reference out"=w151:T6)  [unwired: 5 in]
        n921 = local write "error out"(w148) -> ()
        n922 = Unbundle By Name(w148) -> ("status"=w153:bool)
        n923 = call-poly <vilib>:"PID Control Input Filter.vi"("input"=w149) -> ("output"=w170:dbl)  [unwired: 4 in]
        n924 = case shown="True" w153 {
          tunnel: w169 -> [w186 _]
          tunnel: [w186 w187] -> w175
          frame False {
            n925 = local write "Temperature 2"(w186) -> ()
          }
          frame True {
            n926 = local read "Temperature 2"() -> (w187:dbl)
          }
        }
        n927 = flat-sequence {
          tunnel: w170 -> [w199]
          tunnel: [w199] -> w169
          tunnel: w151 -> [w198]
          tunnel: [w198] -> w150
          frame #0 {
            n928 = Wait (ms)(milliseconds to wait=u32 100) -> ()  [unwired: 1 out]
          }
        }
        n929 = call "IRSensorNIRead.vi"("error in (no error)"=w139, "Melexis_Cmmds"=w136, "Address"=u8 3, "device reference"=w150) -> ("error out"=w141:errorcluster, "Temperature"=w147:dbl, "device reference out"=w146:T6)  [unwired: 5 in]
        n930 = local write "error out"(w141) -> ()
        n931 = Unbundle By Name(w141) -> ("status"=w142:bool)
        n932 = case shown="False" w142 {
          tunnel: w166 -> [w184 _]
          tunnel: [w184 w185] -> w168
          frame False {
            n933 = local write "Temperature 3"(w184) -> ()
          }
          frame True {
            n934 = local read "Temperature 3"() -> (w185:dbl)
          }
        }
        n935 = call-poly <vilib>:"PID Control Input Filter.vi"("input"=w147) -> ("output"=w167:dbl)  [unwired: 4 in]
        n936 = flat-sequence {
          tunnel: w167 -> [w196]
          tunnel: [w196] -> w166
          tunnel: w146 -> [w195]
          tunnel: [w195] -> w144
          frame #0 {
            n937 = Wait (ms)(milliseconds to wait=u32 100) -> ()  [unwired: 1 out]
          }
        }
        n938 = call "IRSensorNIRead.vi"("error in (no error)"=w139, "Melexis_Cmmds"=w136, "Address"=u8 4, "device reference"=w144) -> ("error out"=w131:errorcluster, "Temperature"=w143:dbl, "device reference out"=w138:T6)  [unwired: 5 in]
        n939 = local write "error out"(w131) -> ()
        n940 = Unbundle By Name(w131) -> ("status"=w133:bool)
        n941 = case shown="True" w133 {
          tunnel: w164 -> [w182 _]
          tunnel: [w182 w183] -> w174
          frame False {
            n942 = local write "Temperature 4"(w182) -> ()
          }
          frame True {
            n943 = local read "Temperature 4"() -> (w183:dbl)
          }
        }
        n944 = call-poly <vilib>:"PID Control Input Filter.vi"("input"=w143) -> ("output"=w165:dbl)  [unwired: 4 in]
        n945 = flat-sequence {
          tunnel: w165 -> [w193]
          tunnel: [w193] -> w164
          tunnel: w138 -> [w192]
          tunnel: [w192] -> w137
          frame #0 {
            n946 = Wait (ms)(milliseconds to wait=u32 100) -> ()  [unwired: 1 out]
          }
        }
        n947 = call "IRSensorNIRead.vi"("error in (no error)"=w139, "Melexis_Cmmds"=w136, "Address"=u8 5, "device reference"=w137) -> ("error out"=w134:errorcluster, "Temperature"=w135:dbl)  [unwired: 5 in, 1 out]
        n948 = local write "error out"(w134) -> ()
        n949 = flat-sequence {
          tunnel: w163 -> [w190]
          tunnel: [w190] -> w162
          frame #0 {
            n950 = Wait (ms)(milliseconds to wait=u32 100) -> ()  [unwired: 1 out]
          }
        }
        n951 = Unbundle By Name(w134) -> ("status"=w132:bool)
        n952 = call-poly <vilib>:"PID Control Input Filter.vi"("input"=w135) -> ("output"=w163:dbl)  [unwired: 4 in]
        n953 = local write "error out"(w139) -> ()
        n954 = Build Array(w176, w175, w168, w174, w162) -> (w178:dbl[])
        n955 = Array To Cluster(array=w178) -> (cluster=→"Teperature Chart":T3)
        n956 = case shown="False" w132 {
          tunnel: w162 -> [w180 _]
          tunnel: [w180 w181] -> w173
          frame False {
            n957 = local write "Temperature 5"(w180) -> ()
          }
          frame True {
            n958 = local read "Temperature 5"() -> (w181:dbl)
          }
        }
        n959 = script code="MATLAB script"("T1"=w176, "T2"=w175, "T3"=w168, "T4"=w174, "T5"=w173) -> ()  [unwired: 1 in, 1 out]
      }
      n960 = while {
        stop <- w72 stop-if-true
        n961 = local read "MS task"() -> (w69:refnum<k21>)
        n962 = call-poly <vilib>:"DAQmx Read.vi"("task/channels in"=w69) -> ("data"=w68:dbl[])  [unwired: 12 in, 2 out]
        "MS Array" <- w68
        n963 = script code="MATLAB script"("MS_Data"=w68) -> ()  [unwired: 1 in, 1 out]
        n964 = Build Array(w68) -> (→"MS Signals Chart":dbl[][])
        n965 = Wait (ms)(milliseconds to wait=u32 300) -> ()  [unwired: 1 out]
        n966 = local read "Stop"() -> (w72:bool)
      }
      n967 = while {
        stop <- w94 stop-if-true
        n968 = local read "Pump setpoint(ul/min) 1"() -> (w97:dbl)
        n969 = local read "Pump setpoint(ul/min) 2"() -> (w93:dbl)
        n970 = local read "Pump setpoint(ul/min) 3"() -> (w92:dbl)
        n971 = local read "Pump setpoint(ul/min) 4"() -> (w91:dbl)
        n972 = local read "Pump setpoint(ul/min) 5"() -> (w90:dbl)
        n973 = local read "Pump setpoint(ul/min) 6"() -> (w89:dbl)
        n974 = Build Array(w97, w93, w92, w91, w90, w89) -> (w98:dbl[])
        n975 = Array To Cluster(array=w98) -> (cluster=→"Pump Setpoints Chart":T3)
        n976 = Wait (ms)(milliseconds to wait=u32 5000) -> ()  [unwired: 1 out]
        n977 = local read "Stop"() -> (w94:bool)
      }
      n978 = while {
        stop <- w76 stop-if-true
        n979 = local read "System Error"() -> (w75:bool)
        n980 = Wait (ms)(milliseconds to wait=u32 300) -> ()  [unwired: 1 out]
        n981 = case shown="True" w75 {
          tunnel: [w80 w81] -> w73
          frame False {
            w77 = u16 2 items=["System  Error", "System Running", "System Standby"] ("System Status")
            w78 = u16 1 items=["System  Error", "System Running", "System Standby"] ("System Status")
            n982 = local read "running?"() -> (w79:bool)
            n983 = Select(t=w78, s=w79, f=w77) -> (s? t:f=w80:u16)
          }
          frame True {
            w81 = u16 0 items=["System  Error", "System Running", "System Standby"] ("System Status")
          }
        }
        n984 = local read "Stop"() -> (w76:bool)
        n985 = local write "System Status"(w73) -> ()
      }
      n986 = while {
        tunnel: w62 -> [w82]
        stop <- w88 stop-if-true
        n987 = call-poly <vilib>:"Analog Read.vi"("Analog Channel"=u8 0, "LINX Resource"=w82) -> ("Voltage"=w83:dbl)  [unwired: 6 in, 3 out]
        "Phase_Sensor_voltage" <- w83
        n988 = Wait (ms)(milliseconds to wait=u32 300) -> ()  [unwired: 1 out]
        n989 = Build Array(w83) -> (w85:dbl[])
        n990 = Array To Cluster(array=w85) -> (cluster=→"Phase Sensor Chart":T3)
        n991 = local read "Stop"() -> (w88:bool)
      }
      n992 = while {
        tunnel: w62 -> [w101]
        stop <- w126 stop-if-true
        w108 = 270
        w102 = 600
        w103 = 600
        # "Read Pressure and Flowrate"
        n993 = local read "Stop"() -> (w126:bool)
        n994 = call-poly <vilib>:"Analog Read.vi"("AI Channel(s)"=i32[] [14, 15, 14, 15], "LINX Resource"=w101) -> ("Voltages"=w99:dbl[])  [unwired: 6 in, 3 out]
        n995 = Index Array(array=w99, index=1) -> (element=w122:dbl)
        n996 = Index Array(array=w99, index=0) -> (element=w123:dbl)
        n997 = call-poly <vilib>:"PID Control Input Filter.vi"("input"=w122) -> ("output"=w115:dbl)  [unwired: 4 in]
        n998 = call-poly <vilib>:"PID Control Input Filter.vi"("input"=w123) -> ("output"=w114:dbl)  [unwired: 4 in]
        n999 = Multiply(x=104.96 ("y"), y=w115) -> (x*y=w116:dbl)
        n1000 = Multiply(x=104.96 ("y"), y=w114) -> (x*y=w119:dbl)
        n1001 = Subtract(x=w116, y=24.077) -> (x-y=w106:dbl)
        n1002 = Subtract(x=w119, y=24.077) -> (x-y=w107:dbl)
        n1003 = Build Array(w103, w102) -> (w111:i32[])
        n1004 = Array To Cluster(array=w111) -> (cluster=→"Flowrate Chart":T4)
        n1005 = Build Array(w107, w106) -> (w112:dbl[])
        n1006 = local write "Flowrate Sensor 1"(w103) -> ()
        n1007 = local write "Flowrate Sensor 2"(w102) -> ()
        n1008 = local write "Pressure 1"(w107) -> ()
        n1009 = local write "Pressure 2"(w106) -> ()
        n1010 = Array To Cluster(array=w112) -> (cluster=→"Pressure Chart":T3)
        n1011 = Wait (ms)(milliseconds to wait=u32 500) -> ()  [unwired: 1 out]
        n1012 = script code="MATLAB script"("F1"=w103, "F2"=w102, "Pres1"=w107, "Pres2"=w106) -> ()  [unwired: 1 in, 1 out]
        n1013 = Greater?(x=w106, y=w108) -> (0:w104:bool)
        n1014 = Greater?(x=w107, y=w108) -> (0:w105:bool)
        n1015 = case shown="True" w105 {
          frame False {
          }
          frame True {
            w130 = TRUE ("Stop")
            n1016 = local write "System Error"(w130) -> ()
            n1017 = local write "Stop"(w130) -> ()
            n1018 = local write "Error Message"("Pressure Sensor 1 readings above 250psi") -> ()
            n1019 = script code="system_error = 1;"() -> ()  [unwired: 1 in, 1 out]
          }
        }
        n1020 = case shown="False" w104 {
          frame False {
          }
          frame True {
            w128 = TRUE ("Stop")
            n1021 = local write "System Error"(w128) -> ()
            n1022 = local write "Error Message"("Pressure Sensor 2 readings above 250psi") -> ()
            n1023 = local write "Stop"(w128) -> ()
            n1024 = script code="system_error = 1;"() -> ()  [unwired: 1 in, 1 out]
          }
        }
      }
    }
    frame #3 {
      # "Save and close xml and excel file"
      n1025 = script code="if exist('xl_file','var') & exist('xlApp','var')\n  xlWorkbook.SaveAs(xl_file);\n  xlWorkbook.Close;\n  xlApp.Quit;\n  xlApp.delete;\nend"() -> ()  [unwired: 1 in, 1 out]
    }
    frame #4 {
      w1363 = string[] ["e", "f", "g", "h", "i", "j"]
      # "End communication to hardware"
      n1026 = local read "Syringe_pump?"() -> (w1361:bool)
      n1027 = local read "COMM Port:: Harvard Syringe Pump"() -> (w1362:refnum<visa-resource-name>)
      n1028 = local read "IR Sensor Device"() -> (w1360:T6)
      n1029 = local read "COMM Port :: Milligat Pumps"() -> (w1365:refnum<visa-resource-name>)
      n1030 = call <vilib>:"Close.vi"("LINX Resource"=w1359) -> ()  [unwired: 10 in, 1 out]
      n1031 = Array Size(array=w1363) -> (size(s)=w1364:i32)
      n1032 = case shown="False" w1361 {
        tunnel: w1362 -> [_ w1366]
        frame False {
        }
        frame True {
          n1033 = call <instrlib>:"Stop.vi"("VISA IN"=w1366, "Pump Address"=i8 0) -> ()  [unwired: 7 in, 7 out]
        }
      }
      n1034 = for {
        N: w1364 -> [_]
        tunnel: w1363 -> [w1368] mode=indexing
        tunnel: w1365 -> [w1369]
        n1035 = call "PumpStop.vi"("Pump Address"=w1368, "Pump COMM Port"=w1369) -> ()  [unwired: 9 in, 1 out]
        n1036 = Wait (ms)(milliseconds to wait=u32 300) -> ()  [unwired: 1 out]
      }
      n1037 = call-poly <vilib>:"NI-845x Close Reference.vi"("device reference"=w1360) -> ()  [unwired: 10 in, 1 out]
    }
    frame #5 {
      # "Display Error Messages if necessary"
      n1038 = local read "Error Message"() -> (w1371:string)
      n1039 = One Button Dialog(message=w1371) -> ()  [unwired: 1 in, 1 out]
    }
  }
